vi "SDR_front_panel_V1.vi"() -> ()   [LabVIEW 2024]
uses:
  RPC Messages/rfcontrol_DeviceInformationResponse.ctl
  RPC Messages/rfcontrol_RFDC.ctl
  RPC Messages/rfcontrol_GetRFDCCenterFrequencyResponse.ctl
  RPC Messages/rfcontrol_GetRFDCGainResponse.ctl
  RPC Messages/rfcontrol_RFTile.ctl
  RPC Messages/rfcontrol_GetRFTileSampleRateResponse.ctl
  RPC Messages/rfcontrol_SetRFDCCenterFrequencyResponse.ctl
  RPC Messages/rfcontrol_SetRFDCGainResponse.ctl
  RPC Messages/rfcontrol_SetRFTileSampleRateResponse.ctl
  RPC Messages/rfcontrol_GetRFDCBackgroundCalibrationStateResponse.ctl
  RPC Messages/rfcontrol_SetRFDCBackgroundCalibrationStateResponse.ctl
  RPC Messages/rfcontrol_GetRFDCCalibrationBypassResponse.ctl
  RPC Messages/rfcontrol_SetRFDCCalibrationBypassResponse.ctl
  RPC Messages/rfcontrol_GetDeviceTempsResponse.ctl
  RPC Messages/rfcontrol_TemperatureReadings.ctl
  RPC Messages/rfcontrol_RFDCSendWaveformResponse.ctl
  FlexCompute_grpc_client/RPC Messages/rfcontrol_Response.ctl
  RPC Messages/rfcontrol_SetGPSUTCStartTimeResponse.ctl
  RPC Messages/rfcontrol_RFDCCaptureWaveformRequest.ctl
  RPC Messages/rfcontrol_DeviceInformationRequest.ctl
  RPC Messages/rfcontrol_RFDCSendWaveformRequest.ctl
  RPC Messages/rfcontrol_GetRFDCCenterFrequencyRequest.ctl
  RPC Messages/rfcontrol_GetRFDCGainRequest.ctl
  RPC Messages/rfcontrol_GetRFTileSampleRateRequest.ctl
  RPC Messages/rfcontrol_GetDeviceTempsRequest.ctl
  RPC Messages/rfcontrol_SetRFDCCenterFrequencyRequest.ctl
  RPC Messages/rfcontrol_SetRFDCGainRequest.ctl
  RPC Messages/rfcontrol_SetRFTileSampleRateRequest.ctl
  RPC Messages/rfcontrol_GetRFDCBackgroundCalibrationStateRequest.ctl
  RPC Messages/rfcontrol_SetRFDCBackgroundCalibrationStateRequest.ctl
  RPC Messages/rfcontrol_SetRFDCCalibrationBypassRequest.ctl
  RPC Messages/rfcontrol_GetRFDCCalibrationBypassRequest.ctl
  RPC Messages/rfcontrol_GetTriggerStatusRequest.ctl
  RPC Messages/rfcontrol_SetTriggerWaitRequest.ctl
  RPC Messages/rfcontrol_SetMaxTriggerLengthRequest.ctl
  RPC Messages/rfcontrol_ResetTriggerRequest.ctl
  RPC Messages/rfcontrol_StartGPSPollRequest.ctl
  RPC Messages/rfcontrol_StopGPSPollRequest.ctl
  RPC Messages/rfcontrol_SetGPSUTCStartTimeRequest.ctl
  FlexCompute_grpc_client/RPC Messages/rfcontrol_ControlParams.ctl
  FlexCompute_grpc_client/RPC Messages/rfcontrol_Empty.ctl
  RPC Messages/rfcontrol_GetGPSLastLocInfoRequest.ctl
  FlexSDR_gRPC_client.lvlib
  FlexCompute_grpc_client/FlexCompute_grpc_client.lvlib
panel:
  in  "FlexCompute Selection":u16(ring) items=["192.168.137.105:5555"]
  out "Error Out":errorcluster
  in  "Clear\nDevices":bool
  out "FlexSDR Search IP":string
  in  "FlexSDR Search Subnet":string
  in  "FlexSDR Selection":u16(ring) items=["192.168.137.76:5555", "192.168.137.105:5555", "192.168.137.173:5555", "192.168.137.174:5555"]
  in  "Scan for \nDevices":bool
  out "Hardware\nBusy":bool
  in  "Stop Program":bool
  in  "Main Container":T1(tab)
  in  "Set Default Scale":bool
  in  "Continuous I/Q Capture":bool
  in  "WFM Type":string(combo)
  in  "Send RFDC":T2
  in  "Set TX Waveform":bool
  out "Capture Error Status":i32
  out "Capture Error Message":string
  out "IQ Graph":cluster{"Y":dbl[], "Y":dbl[]}[](graph)
  in  "Capture Length":i32
  in  "Capture RFDC":T2
  in  "Single I/Q Capture":bool
  out "Send WFM Resp":T3
  out "FFT Mag":cluster{"Y":dbl[], "Y":dbl[]}[](graph)
  in  "Get Gain":bool
  in  "Gain RFDC":T2
  in  "Get Center\nFrequency":bool
  in  "Get Device\nInformation":bool
  out "Device\nInformation":T4
  in  "CF RFDC":T2
  out "Center Frequency Data":T5 {"center_frequency" format="%#_g MHz"}
  out "Gain Data":T6 {"gain" format="%#_g dB"}
  in  "Get Sample\nRate":bool
  in  "SR RFTile":T7
  out "Sample Rate Data":T8 {"sample_rate" format="%#_g MSps"}
  out "Device Temp Data":T9 {"temp_readings"."RPU_temp" format="%#_g °C"; "temp_readings"."APU_temp" format="%#_g °C"; "temp_readings"."PL_temp" format="%#_g °C"}
  in  "Get Temps":bool
  in  "Req SR":dbl format="%#_g MSps"
  in  "Set Sample\nRate":bool
  in  "SSR RFTile":T7
  in  "Set Gain":bool
  in  "SG RFDC":T2
  in  "Req Gain":dbl format="%#_g dB"
  in  "Set Center\nFrequency":bool
  in  "SCF RFDC":T2
  out "SCF Data":T11 {"center_frequency" format="%#_g MHz"}
  in  "Req CF":dbl format="%#_g MHz"
  out "SG Data":T12 {"gain" format="%#_g dB"}
  out "SSR Data":T13 {"sample_rate" format="%#_g MSps"}
  out "Analyzing\n100 MHz":bool
  out "Grabbing\n100 MHz":bool
  out "Analyzing\n400 MHz":bool
  out "Grabbing\n400 MHz":bool
  out "Analyzing\n1200 MHz":bool
  out "Grabbing\n1200 MHz":bool
  in  "Cal Level":dbl format="%#_g dBm"
  in  "Show Matlab":bool
  out "Writing \nCal Coeffs":bool
  out "100 EVM":dbl format="%#_g dB"
  out "400 EVM":dbl format="%#_g dB"
  out "1200 EVM":dbl format="%#_g dB"
  out "Complete":bool
  out "Analyzing\nFull BW":bool
  out "Grabbing\nFull BW":bool
  out "Cal FFT Mag":cluster{"Y":dbl[], "Y":dbl[]}[](graph)
  in  "Perform CAL":bool
  out "Full BW EVM":dbl format="%#_g dB"
  in  "New Cal Status":bool
  in  "SBCal RFDC":T2
  in  "Set Cal\nStatus":bool
  in  "Cal RFDC":T2
  in  "Get Cal\nStatus":bool
  in  "New Frozen\nStatus":bool
  in  "SBGCal RFDC":T2
  in  "Set BGCal\nStatus":bool
  in  "BGCal RFDC":T2
  in  "Get BGCal\nStatus":bool
  out "BGCal Data":T14
  out "SBGCal Data":T15
  out "Cal Status Data":T16
  out "SCal Status Data":T17
  out "Set Trig Max Length Error Status":i32
  out "Set Trig Max Length Error Message":string
  in  "Set Trig Max Length":bool
  out "Reset Trig Error Status":i32
  out "Reset Trig Error Message":string
  in  "Reset Trig":bool
  out "Set Trig Wait Error Status":i32
  out "Set Trig Wait Error Message":string
  in  "Set Hardware Trig":bool
  in  "Set Trig Max Length Value":i32 format="%.0f Samples"
  in  "Set Trig Delay":i32 format="%.0f Samples"
  in  "Set Trig Wait":bool
  out "Get Trig Status Error Status":i32
  out "Get Trig Status Error Message":string
  out "Hardware Trig?":bool
  out "Wait For Trig?":bool
  out "Triggered?":bool
  in  "Get Trig\nStatus":bool
  in  "Channel #":i32
  in  "Quad #":i32
  out "Trig Delay":i32 format="%.0f Samples"
  out "Trig Max Length":i32 format="%.0f Samples"
  in  "Display \nTimestamp?":bool
  in  "UTC Start Time":dbl format="%#_12g"
  in  "Set UTC\nStart Time":bool
  in  "GPS Num of Samples":i32(ring) items=["1 Sample"=1, "2 Samples"=2, "3 Samples"=3, "4 Samples"=4, "5 Samples"=5]
  out "GPS Poll Active":bool
  in  "Start GPS \nPoll":bool
  in  "Stop GPS\nPoll":bool
  in  "GPS Poll Time":dbl format="%#_g ms"
  out "GPS Actual Poll Time":u32 format="%.0f ms"
  out "GPS ECEF Y":dbl[](array[numeric]) format="%#_9g"
  out "GPS ECEF X":dbl[](array[numeric]) format="%#_9f"
  out "GPS ECEF Z":dbl[](array[numeric]) format="%#_9g"
  out "GPS error_status":i32
  out "GPS error_message":string
  out "GPS Time":string[](array[string])
  out "UTS Start Time Response":T18 {"utc_start_time" format="%#_12g"}
  in  "Set Peak Threshold":dbl format="%#_g dBm"
  in  "Update Server\nControls":bool
  out "KPI Error Message":string
  out "KPI Status":u32
  out "Mem Address":string
  out "Anomaly \nDetected":bool
  out "RSSI":dbl format="%#_g dBm"
  out "Actual KPI Poll Time":u32 format="%.0f ms"
  in  "KPI Poll":bool
  in  "KPI Poll Time":dbl format="%#_g ms"
  out "I Phase Rotation From Peak":dbl format="%#_g Hz"
  out "Peak Time Offset":dbl format="%#_g ns"
  out "Q Phase Rotation From Peak":dbl format="%#_g Hz"
  out "Peak Threshold":dbl format="%#_g dBm"
  out "Peak Time":dbl format="%#_g s"
  in  "Set Server Sample Rate":dbl format="%#_g MHz"
  in  "Set Carrier Frequency":dbl format="%#_g MHz"
  in  "Set Sync Length":i32 format="%.0f Samples"
  in  "Set Time Between Peaks":dbl format="%#_g µs"
  out "Update Server Controls Response":T19
  # "Tile Mapping:\n\nTXT1:\n1. TX1     2. TX2\n3. TX3     4. TX4\n\nTXT2:\n1. TX5     2. TX6\n3. TX7     4. TX8\n\nRXT1:\n1. RX1     2. RX2\n3. RX3     4. RX4\n\nRXT2:\n1. RX5     2. RX6\n3. RX7     4. RX8\n\nWRXT:\n1. WRX1   2.WRX2"
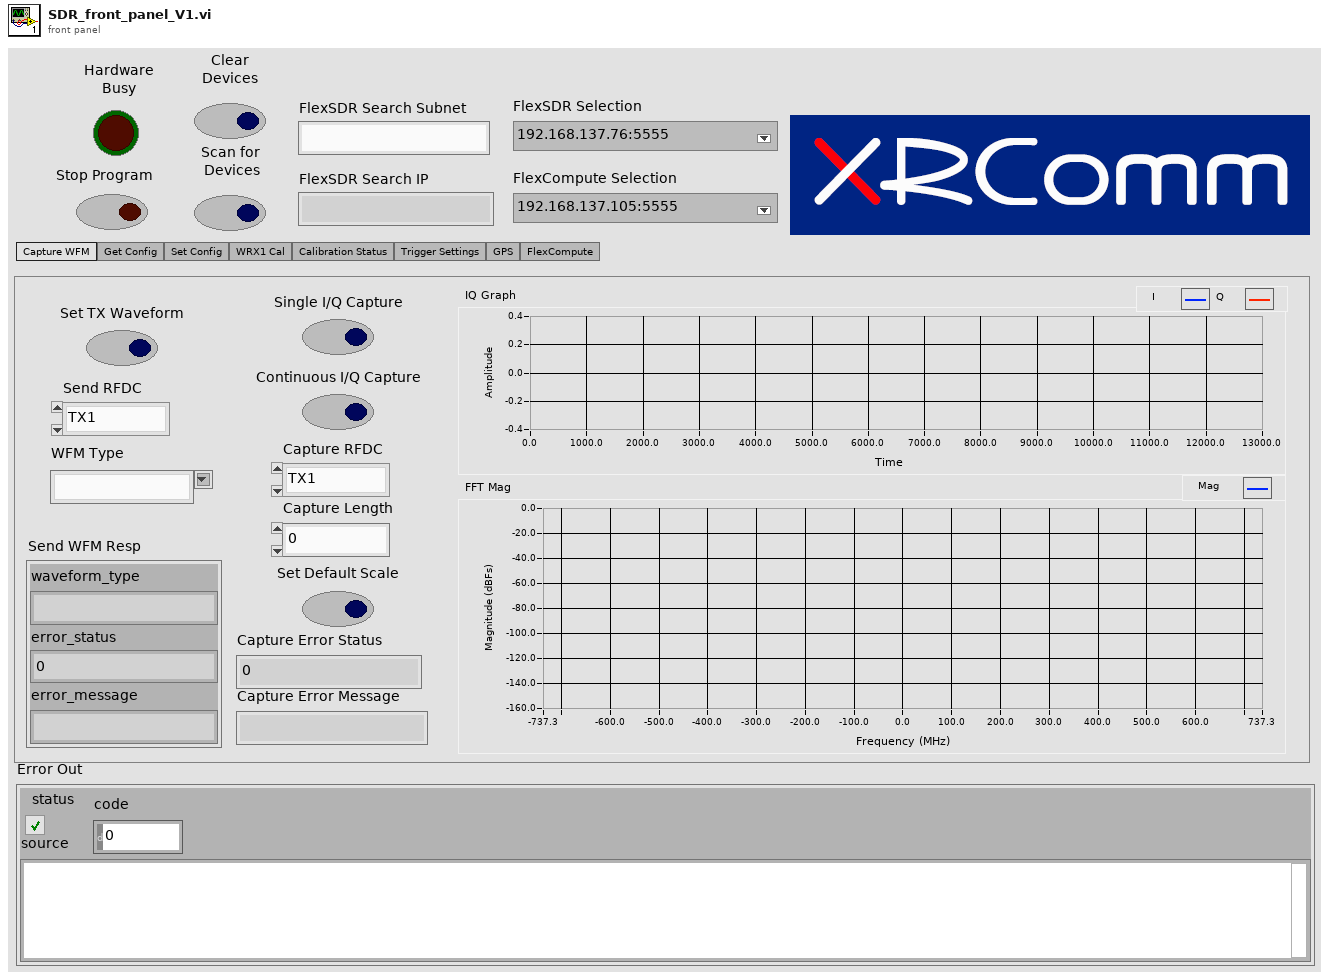
[diagram p1: front panel]
types:
  T1 = enum32{"Capture WFM", "Get Config", "Set Config", "WRX1 Cal", "Calibration Status", "Trigger Settings", "GPS", "FlexCompute"}
  T2 = typedef "FlexSDR_gRPC_client.lvlib/rfcontrol_RFDC.ctl" = enum32{"TX1", "TX2", "TX3", "TX4", "TX5", "TX6", "TX7", "TX8", "RX1", "RX2", "RX3", "RX4", "RX5", "RX6", "RX7", "RX8", "WRX1", "WRX2"}
  T3 = typedef "FlexSDR_gRPC_client.lvlib/rfcontrol_RFDCSendWaveformResponse.ctl" = cluster{"waveform_type":string, "error_status":i32, "error_message":string}
  T4 = typedef "FlexSDR_gRPC_client.lvlib/rfcontrol_DeviceInformationResponse.ctl" = cluster{"reply_information":string, "manufacturer":string, "model":string, "serial_number":i32, "firmware_revision":string}
  T5 = typedef "FlexSDR_gRPC_client.lvlib/rfcontrol_GetRFDCCenterFrequencyResponse.ctl" = cluster{"center_frequency":dbl, "error_status":i32, "error_message":string}
  T6 = typedef "FlexSDR_gRPC_client.lvlib/rfcontrol_GetRFDCGainResponse.ctl" = cluster{"gain":dbl, "error_status":i32, "error_message":string}
  T7 = typedef "FlexSDR_gRPC_client.lvlib/rfcontrol_RFTile.ctl" = enum32{"TXT1", "TXT2", "RXT1", "RXT2", "WRXT"}
  T8 = typedef "FlexSDR_gRPC_client.lvlib/rfcontrol_GetRFTileSampleRateResponse.ctl" = cluster{"sample_rate":dbl, "error_status":i32, "error_message":string}
  T9 = typedef "FlexSDR_gRPC_client.lvlib/rfcontrol_GetDeviceTempsResponse.ctl" = cluster{"temp_readings":T10, "error_status":i32, "error_message":string}
  T10 = typedef "FlexSDR_gRPC_client.lvlib/rfcontrol_TemperatureReadings.ctl" = cluster{"PL_temp":dbl, "APU_temp":dbl, "RPU_temp":dbl}
  T11 = typedef "FlexSDR_gRPC_client.lvlib/rfcontrol_SetRFDCCenterFrequencyResponse.ctl" = cluster{"center_frequency":dbl, "error_status":i32, "error_message":string}
  T12 = typedef "FlexSDR_gRPC_client.lvlib/rfcontrol_SetRFDCGainResponse.ctl" = cluster{"gain":dbl, "error_status":i32, "error_message":string}
  T13 = typedef "FlexSDR_gRPC_client.lvlib/rfcontrol_SetRFTileSampleRateResponse.ctl" = cluster{"sample_rate":dbl, "error_status":i32, "error_message":string}
  T14 = typedef "FlexSDR_gRPC_client.lvlib/rfcontrol_GetRFDCBackgroundCalibrationStateResponse.ctl" = cluster{"is_frozen":bool, "error_status":i32, "error_message":string}
  T15 = typedef "FlexSDR_gRPC_client.lvlib/rfcontrol_SetRFDCBackgroundCalibrationStateResponse.ctl" = cluster{"is_frozen":bool, "error_status":i32, "error_message":string}
  T16 = typedef "FlexSDR_gRPC_client.lvlib/rfcontrol_GetRFDCCalibrationBypassResponse.ctl" = cluster{"bypass_cal":bool, "error_status":i32, "error_message":string}
  T17 = typedef "FlexSDR_gRPC_client.lvlib/rfcontrol_SetRFDCCalibrationBypassResponse.ctl" = cluster{"bypass_cal":bool, "error_status":i32, "error_message":string}
  T18 = typedef "FlexSDR_gRPC_client.lvlib/rfcontrol_SetGPSUTCStartTimeResponse.ctl" = cluster{"utc_start_time":dbl, "error_status":i32, "error_message":string}
  T19 = typedef "FlexCompute_grpc_client.lvlib/rfcontrol_Response.ctl" = cluster{"message":string}
  T20 = enum8{"Enabled", "Disabled", "Disabled and Grayed Out"}
  T21 = typedef "FlexCompute_grpc_client.lvlib/rfcontrol_Empty.ctl" = cluster{"void":string}
  T22 = typedef "FlexSDR_gRPC_client.lvlib/rfcontrol_RFDCCaptureWaveformRequest.ctl" = cluster{"device_id":string, "rfdc":T2, "num_of_samples":i32, "error_queue_populate":bool}
  T23 = typedef "FlexSDR_gRPC_client.lvlib/rfcontrol_GetGPSLastLocInfoRequest.ctl" = cluster{"device_id":string, "num_of_samples":i32, "error_queue_populate":bool}
  T24 = typedef "FlexSDR_gRPC_client.lvlib/rfcontrol_DeviceInformationRequest.ctl" = cluster{"device_id":string, "error_queue_populate":bool}
  T25 = typedef "FlexSDR_gRPC_client.lvlib/rfcontrol_RFDCSendWaveformRequest.ctl" = cluster{"device_id":string, "rfdc":T2, "waveform_type":string, "error_queue_populate":bool}
  T26 = typedef "FlexSDR_gRPC_client.lvlib/rfcontrol_GetRFDCCenterFrequencyRequest.ctl" = cluster{"device_id":string, "rfdc":T2, "error_queue_populate":bool}
  T27 = typedef "FlexSDR_gRPC_client.lvlib/rfcontrol_GetRFDCGainRequest.ctl" = cluster{"device_id":string, "rfdc":T2, "error_queue_populate":bool}
  T28 = typedef "FlexSDR_gRPC_client.lvlib/rfcontrol_GetRFTileSampleRateRequest.ctl" = cluster{"device_id":string, "rftile":T7, "error_queue_populate":bool}
  T29 = typedef "FlexSDR_gRPC_client.lvlib/rfcontrol_GetDeviceTempsRequest.ctl" = cluster{"device_id":string, "error_queue_populate":bool}
  T30 = typedef "FlexSDR_gRPC_client.lvlib/rfcontrol_SetRFDCCenterFrequencyRequest.ctl" = cluster{"device_id":string, "rfdc":T2, "center_frequency":dbl, "error_queue_populate":bool}
  T31 = typedef "FlexSDR_gRPC_client.lvlib/rfcontrol_SetRFDCGainRequest.ctl" = cluster{"device_id":string, "rfdc":T2, "gain":dbl, "error_queue_populate":bool}
  T32 = typedef "FlexSDR_gRPC_client.lvlib/rfcontrol_SetRFTileSampleRateRequest.ctl" = cluster{"device_id":string, "rftile":T7, "sample_rate":dbl, "error_queue_populate":bool}
  T33 = typedef "FlexSDR_gRPC_client.lvlib/rfcontrol_SetRFDCCalibrationBypassRequest.ctl" = cluster{"device_id":string, "rfdc":T2, "bypass_cal":bool, "error_queue_populate":bool}
  T34 = typedef "FlexSDR_gRPC_client.lvlib/rfcontrol_SetRFDCBackgroundCalibrationStateRequest.ctl" = cluster{"device_id":string, "rfdc":T2, "is_frozen":bool, "error_queue_populate":bool}
  T35 = typedef "FlexSDR_gRPC_client.lvlib/rfcontrol_GetRFDCBackgroundCalibrationStateRequest.ctl" = cluster{"device_id":string, "rfdc":T2, "error_queue_populate":bool}
  T36 = typedef "FlexSDR_gRPC_client.lvlib/rfcontrol_GetRFDCCalibrationBypassRequest.ctl" = cluster{"device_id":string, "rfdc":T2, "error_queue_populate":bool}
  T37 = typedef "FlexSDR_gRPC_client.lvlib/rfcontrol_GetTriggerStatusRequest.ctl" = cluster{"device_id":string, "quad_num":i32, "channel_num":i32, "error_queue_populate":bool}
  T38 = typedef "FlexSDR_gRPC_client.lvlib/rfcontrol_SetTriggerWaitRequest.ctl" = cluster{"device_id":string, "quad_num":i32, "channel_num":i32, "trig_sample_delay":i32, "is_hardware_trig":bool, "error_queue_populate":bool}
  T39 = typedef "FlexSDR_gRPC_client.lvlib/rfcontrol_SetMaxTriggerLengthRequest.ctl" = cluster{"device_id":string, "quad_num":i32, "channel_num":i32, "max_trig_length":i32, "error_queue_populate":bool}
  T40 = typedef "FlexSDR_gRPC_client.lvlib/rfcontrol_ResetTriggerRequest.ctl" = cluster{"device_id":string, "quad_num":i32, "channel_num":i32, "error_queue_populate":bool}
  T41 = typedef "FlexSDR_gRPC_client.lvlib/rfcontrol_StartGPSPollRequest.ctl" = cluster{"device_id":string, "error_queue_populate":bool}
  T42 = typedef "FlexSDR_gRPC_client.lvlib/rfcontrol_StopGPSPollRequest.ctl" = cluster{"device_id":string, "error_queue_populate":bool}
  T43 = typedef "FlexSDR_gRPC_client.lvlib/rfcontrol_SetGPSUTCStartTimeRequest.ctl" = cluster{"device_id":string, "utc_start_time":dbl, "error_queue_populate":bool}
  T44 = typedef "FlexCompute_grpc_client.lvlib/rfcontrol_ControlParams.ctl" = cluster{"peak_threshold":dbl, "sampling_rate_hz":dbl, "carrier_frequency_hz":dbl, "sync_length_samples":u32, "time_between_peaks_s":dbl}
  T45 = typedef "grpc-lvsupport-release.lvlib/grpcId.ctl" = u64
  T46 = typedef "FlexSDR_gRPC_client.lvlib/rfcontrol_RFDCCaptureWaveformResponse.ctl" = cluster{"I":dbl[], "Q":dbl[], "error_status":i32, "error_message":string}
  T47 = typedef "FlexSDR_gRPC_client.lvlib/rfcontrol_GetTriggerStatusResponse.ctl" = cluster{"quad_num":i32, "channel_num":i32, "triggered":bool, "wait_for_trig":bool, "trig_sample_delay":i32, "is_hardware_trig":bool, "max_trig_length":i32, "error_status":i32, "error_message":string}
  T48 = typedef "FlexSDR_gRPC_client.lvlib/rfcontrol_SetTriggerWaitResponse.ctl" = cluster{"quad_num":i32, "channel_num":i32, "trig_sample_delay":i32, "is_hardware_trig":bool, "error_status":i32, "error_message":string}
  T49 = typedef "FlexSDR_gRPC_client.lvlib/rfcontrol_SetMaxTriggerLengthResponse.ctl" = cluster{"quad_num":i32, "channel_num":i32, "max_trig_length":i32, "error_status":i32, "error_message":string}
  T50 = typedef "FlexSDR_gRPC_client.lvlib/rfcontrol_ResetTriggerResponse.ctl" = cluster{"quad_num":i32, "channel_num":i32, "error_status":i32, "error_message":string}
  T51 = typedef "FlexSDR_gRPC_client.lvlib/rfcontrol_StartGPSPollResponse.ctl" = cluster{"gps_poll_status":bool, "error_status":i32, "error_message":string}
  T52 = typedef "FlexSDR_gRPC_client.lvlib/rfcontrol_StopGPSPollResponse.ctl" = cluster{"gps_poll_status":bool, "error_status":i32, "error_message":string}
  T53 = typedef "FlexSDR_gRPC_client.lvlib/rfcontrol_GetGPSLastLocInfoResponse.ctl" = cluster{"time":dbl[], "ecef_x":dbl[], "ecef_y":dbl[], "ecef_z":dbl[], "error_status":i32, "error_message":string}
  T54 = typedef "FlexCompute_grpc_client.lvlib/rfcontrol_KPIData.ctl" = cluster{"peak_threshold":dbl, "rssi_db":dbl, "timing_offset_s":dbl, "peak_index_samples":i32, "peak_time_s":dbl, "is_anomaly":bool, "mem_address":string, "status":T55, "error_message":string, "phase_rotation_from_peak_I":sgl, "phase_rotation_from_peak_Q":sgl}
  T55 = typedef "FlexCompute_grpc_client.lvlib/rfcontrol_Status.ctl" = enum32{"SUCCESS", "ERROR"}
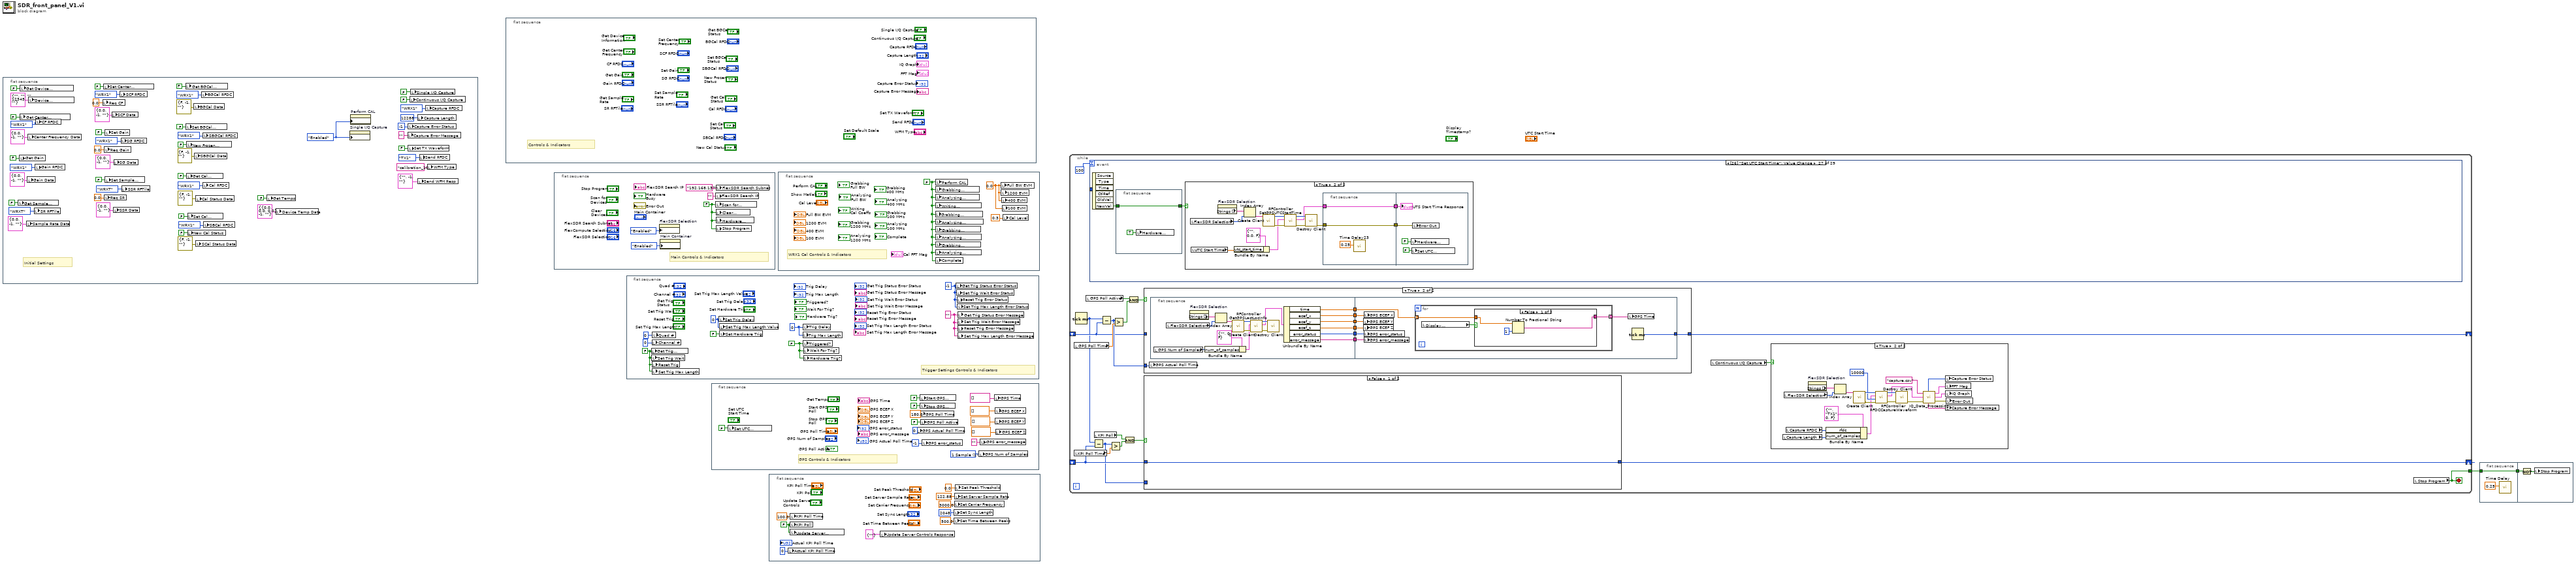
[diagram p0: block diagram]
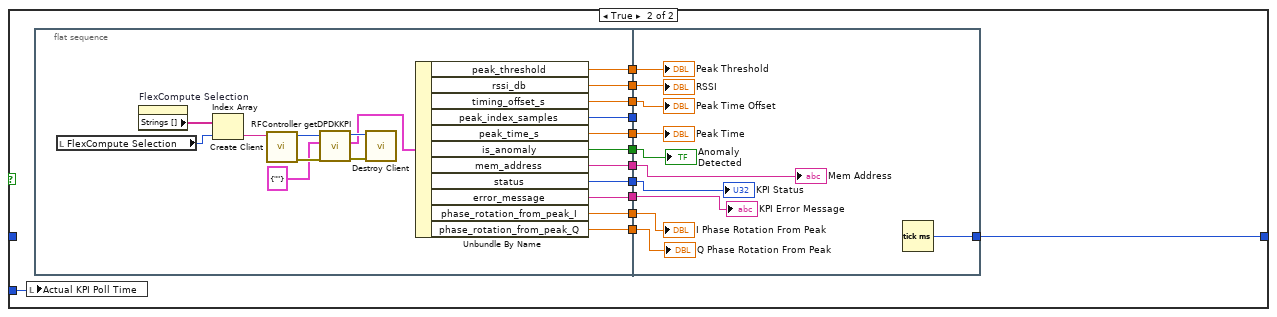
[diagram p2: hidden frame]
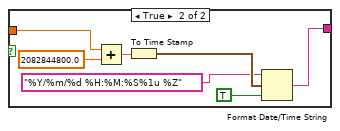
[diagram p5: hidden frame]
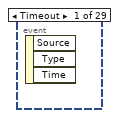
[diagram p6: hidden frame]
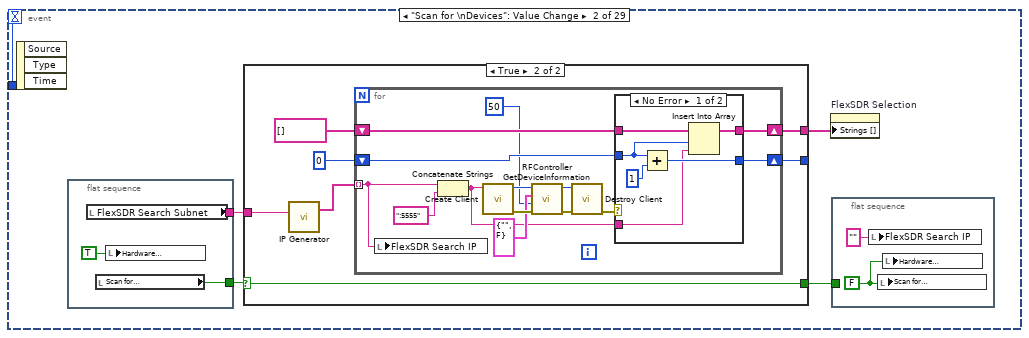
[diagram p7: hidden frame]
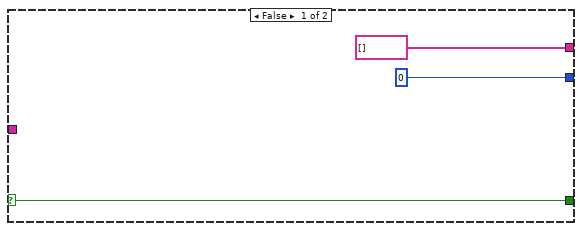
[diagram p8: hidden frame]
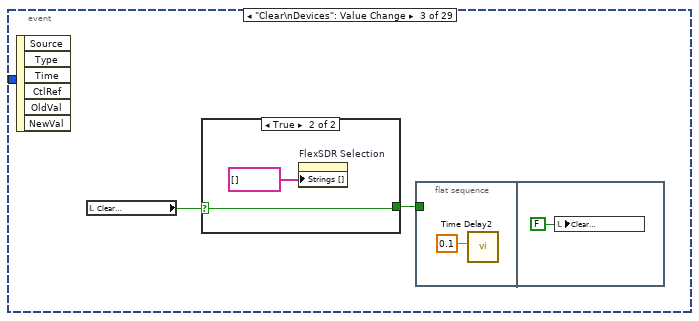
[diagram p10: hidden frame]
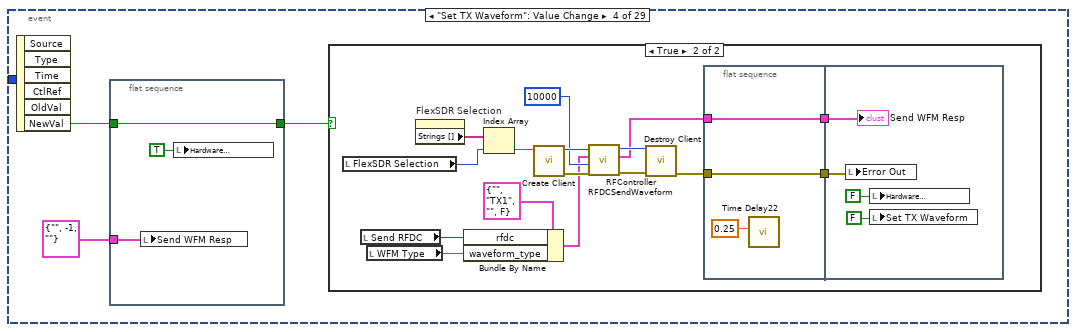
[diagram p12: hidden frame]
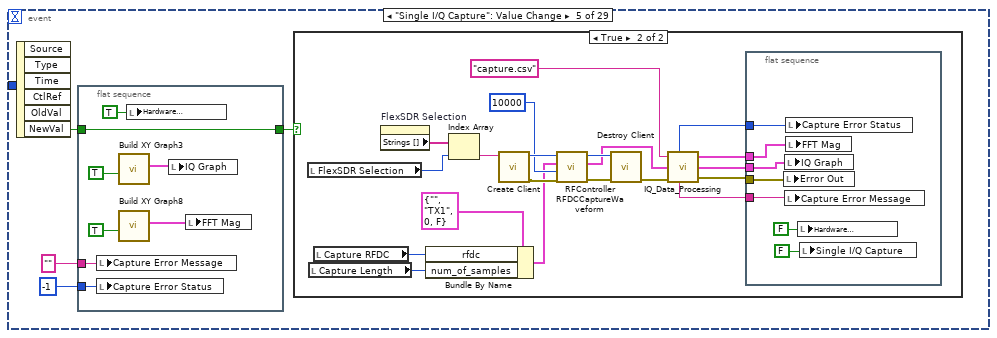
[diagram p14: hidden frame]
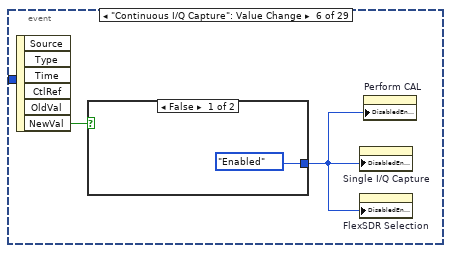
[diagram p16: hidden frame]
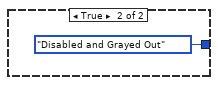
[diagram p17: hidden frame]
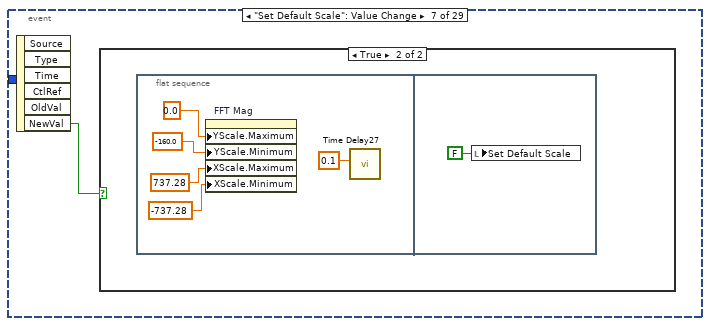
[diagram p18: hidden frame]
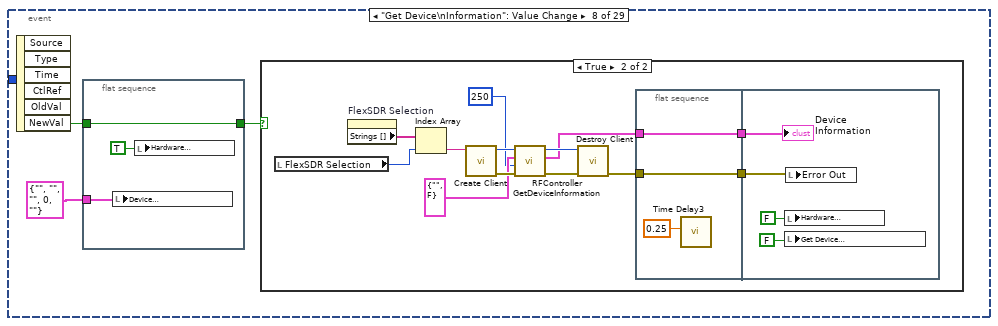
[diagram p20: hidden frame]
diagram:
  n1 = flat-sequence {
    frame #0 {
      w3 = T20."Enabled" ("Disabled")
      # "Initial Settings"
      n2 = local write "Get Sample\nRate"(FALSE ("Get Sample\nRate")) -> ()
      n3 = local write "Get Gain"(FALSE ("Get Gain")) -> ()
      n4 = local write "Get Center\nFrequency"(FALSE ("Get Center\nFrequency")) -> ()
      n5 = local write "Get Device\nInformation"(FALSE ("Get Device\nInformation")) -> ()
      n6 = local write "Sample Rate Data"(T8 {"sample_rate"=0.0, "error_status"=-1, "error_message"=""} ("Sample Rate Data")) -> ()
      n7 = local write "Gain Data"(T6 {"gain"=0.0, "error_status"=-1, "error_message"=""} ("Gain Data")) -> ()
      n8 = local write "Center Frequency Data"(T5 {"center_frequency"=0.0, "error_status"=-1, "error_message"=""} ("Center Frequency Data")) -> ()
      n9 = local write "Device\nInformation"(T4 {"reply_information"="", "manufacturer"="", "model"="", "serial_number"=12345, "firmware_revision"=""} ("Device\nInformation")) -> ()
      n10 = local write "SR RFTile"(rfcontrol_RFTile."WRXT" ("SR RFTile")) -> ()
      n11 = local write "Gain RFDC"(rfcontrol_RFDC."WRX1" ("Gain RFDC")) -> ()
      n12 = local write "CF RFDC"(rfcontrol_RFDC."WRX1" ("CF RFDC")) -> ()
      n13 = local write "Req CF"(0.0 ("Req CF")) -> ()
      n14 = local write "Set Center\nFrequency"(FALSE ("Set Center\nFrequency")) -> ()
      n15 = local write "Req Gain"(0.0 ("Req Gain")) -> ()
      n16 = local write "Req SR"(0.0 ("Req SR")) -> ()
      n17 = local write "Set Gain"(FALSE ("Set Gain")) -> ()
      n18 = local write "Set Sample\nRate"(FALSE ("Set Sample\nRate")) -> ()
      n19 = local write "SCF Data"(T11 {"center_frequency"=0.0, "error_status"=-1, "error_message"=""} ("Response Data")) -> ()
      n20 = local write "SSR Data"(T13 {"sample_rate"=0.0, "error_status"=-1, "error_message"=""} ("SSR Data")) -> ()
      n21 = local write "SG Data"(T12 {"gain"=0.0, "error_status"=-1, "error_message"=""} ("SG Data")) -> ()
      n22 = local write "SCF RFDC"(rfcontrol_RFDC."WRX1" ("SCF RFDC")) -> ()
      n23 = local write "SG RFDC"(rfcontrol_RFDC."WRX1" ("SG RFDC")) -> ()
      n24 = local write "SSR RFTile"(rfcontrol_RFTile."WRXT" ("SSR Tile")) -> ()
      n25 = local write "Get BGCal\nStatus"(FALSE ("Get BGCal\nStatus")) -> ()
      n26 = local write "Set BGCal\nStatus"(FALSE ("Set BGCal\nStatus")) -> ()
      n27 = local write "New Frozen\nStatus"(FALSE ("New Frozen\nStatus")) -> ()
      n28 = local write "Get Cal\nStatus"(FALSE ("Get Cal\nStatus")) -> ()
      n29 = local write "Set Cal\nStatus"(FALSE ("Set Cal\nStatus")) -> ()
      n30 = local write "New Cal Status"(FALSE ("New Cal Status")) -> ()
      n31 = local write "BGCal Data"(T14 {"is_frozen"=FALSE, "error_status"=-1, "error_message"=""} ("BGCal Data")) -> ()
      n32 = local write "SBGCal Data"(T15 {"is_frozen"=FALSE, "error_status"=-1, "error_message"=""} ("SBGCal Data")) -> ()
      n33 = local write "SCal Status Data"(T17 {"bypass_cal"=FALSE, "error_status"=-1, "error_message"=""} ("SCal Status Data")) -> ()
      n34 = local write "Cal Status Data"(T16 {"bypass_cal"=FALSE, "error_status"=-1, "error_message"=""} ("Cal Status Data")) -> ()
      n35 = local write "BGCal RFDC"(rfcontrol_RFDC."WRX1" ("BGCal RFDC")) -> ()
      n36 = local write "SBGCal RFDC"(rfcontrol_RFDC."WRX1" ("SBGCal RFDC")) -> ()
      n37 = local write "Cal RFDC"(rfcontrol_RFDC."WRX1" ("Cal RFDC")) -> ()
      n38 = local write "SBCal RFDC"(rfcontrol_RFDC."WRX1" ("SBCal RFDC")) -> ()
      n39 = local write "Get Temps"(FALSE ("Get Temps")) -> ()
      n40 = local write "Device Temp Data"(T9 {"temp_readings"={"PL_temp"=0.0, "APU_temp"=0.0, "RPU_temp"=0.0}, "error_status"=-1, "error_message"=""} ("Device Temp Data")) -> ()
      n41 = property on="Single I/Q Capture" class="Bool (strict)"("DisabledEnum"=w3) -> ()  [unwired: 2 in, 2 out]
      n42 = property on="Perform CAL" class="Bool (strict)"("DisabledEnum"=w3) -> ()  [unwired: 2 in, 2 out]
      n43 = local write "Capture Error Message"("" ("Capture Error Message")) -> ()
      n44 = local write "Capture Error Status"(-1 ("Capture Error Status")) -> ()
      n45 = local write "Set TX Waveform"(FALSE ("Set TX Waveform")) -> ()
      n46 = local write "Continuous I/Q Capture"(FALSE ("Continuous I/Q Capture")) -> ()
      n47 = local write "Single I/Q Capture"(FALSE ("Grab I/Q Waveform")) -> ()
      n48 = local write "Capture Length"(12288 ("Capture Length")) -> ()
      n49 = local write "Send WFM Resp"(T3 {"waveform_type"="", "error_status"=-1, "error_message"=""} ("Send WFM Resp")) -> ()
      n50 = local write "Send RFDC"(rfcontrol_RFDC."TX1" ("Send RFDC")) -> ()
      n51 = local write "Capture RFDC"(rfcontrol_RFDC."WRX1" ("Capture RFDC")) -> ()
      n52 = local write "WFM Type"("calibration_100" ("WFM Type")) -> ()
    }
  }
  n53 = flat-sequence {
    frame #0 {
      # "Controls & Indicators"
    }
  }
  n54 = flat-sequence {
    frame #0 {
      w55 = FALSE ("Scan for \nDevices")
      # "Main Controls & Indicators"
      n55 = property on="FlexSDR Selection" class="Ring (strict)"("DisabledEnum"=T20."Enabled" ("Disabled")) -> ()  [unwired: 2 in, 2 out]
      n56 = property on="Main Container" class="TabCtl (strict)"("DisabledEnum"=T20."Enabled" ("Disabled")) -> ()  [unwired: 2 in, 2 out]
      n57 = local write "FlexSDR Search IP"("" ("Current Search IP")) -> ()
      n58 = local write "Scan for \nDevices"(w55) -> ()
      n59 = local write "FlexSDR Search Subnet"("192.168.137" ("Search Subnet")) -> ()
      n60 = local write "Clear\nDevices"(w55) -> ()
      n61 = local write "Hardware\nBusy"(w55) -> ()
      n62 = local write "Stop Program"(w55) -> ()
    }
  }
  n63 = flat-sequence {
    frame #0 {
      w60 = "" ("Set Trig Wait Error Message")
      w61 = -1 ("Set Trig Wait Error Status")
      w59 = 0 ("Set Trig Delay")
      w63 = 0 ("Trig Delay")
      w64 = FALSE ("Triggered?")
      w58 = FALSE ("Get Trig\nStatus")
      # "Trigger Settings Controls & Indicators"
      n64 = local write "Get Trig\nStatus"(w58) -> ()
      n65 = local write "Set Trig Wait"(w58) -> ()
      n66 = local write "Channel #"(0 ("Channel #")) -> ()
      n67 = local write "Reset Trig"(w58) -> ()
      n68 = local write "Set Trig Max Length"(w58) -> ()
      n69 = local write "Quad #"(0 ("Quad #")) -> ()
      n70 = local write "Set Trig Delay"(w59) -> ()
      n71 = local write "Set Trig Max Length Value"(w59) -> ()
      n72 = local write "Set Hardware Trig"(FALSE ("Set Hardware Trig")) -> ()
      n73 = local write "Trig Max Length"(w63) -> ()
      n74 = local write "Trig Delay"(w63) -> ()
      n75 = local write "Triggered?"(w64) -> ()
      n76 = local write "Wait For Trig?"(w64) -> ()
      n77 = local write "Hardware Trig?"(w64) -> ()
      n78 = local write "Get Trig Status Error Status"(w61) -> ()
      n79 = local write "Set Trig Wait Error Status"(w61) -> ()
      n80 = local write "Reset Trig Error Status"(w61) -> ()
      n81 = local write "Set Trig Max Length Error Status"(w61) -> ()
      n82 = local write "Get Trig Status Error Message"(w60) -> ()
      n83 = local write "Set Trig Wait Error Message"(w60) -> ()
      n84 = local write "Reset Trig Error Message"(w60) -> ()
      n85 = local write "Set Trig Max Length Error Message"(w60) -> ()
    }
  }
  n86 = flat-sequence {
    frame #0 {
      w68 = 1 items=["1 Sample"=1, "2 Samples"=2, "3 Samples"=3, "4 Samples"=4, "5 Samples"=5] ("GPS Num of Samples")
      # "GPS Controls & Indicators"
      n87 = local write "Set UTC\nStart Time"(FALSE ("Set UTC\nStart Time")) -> ()
      n88 = local write "GPS Actual Poll Time"(u32 0 ("Actual Poll Time")) -> ()
      n89 = local write "GPS Poll Time"(180.0 ("Poll Time")) -> ()
      n90 = local write "Start GPS \nPoll"(FALSE ("Start GPS \nPoll")) -> ()
      n91 = local write "Stop GPS\nPoll"(FALSE ("Stop GPS\nPoll")) -> ()
      n92 = local write "GPS Poll Active"(FALSE ("GPS Poll Active")) -> ()
      n93 = local write "GPS error_status"(-1 ("GPS error_status")) -> ()
      n94 = local write "GPS Num of Samples"(w68) -> ()
      n95 = local write "GPS error_message"("" ("GPS error_message")) -> ()
      n96 = local write "GPS Time"(string[] [] ("GPS Time")) -> ()
      n97 = local write "GPS ECEF X"(dbl[] [] ("ecef_x")) -> ()
      n98 = local write "GPS ECEF Y"(dbl[] [] ("ecef_y")) -> ()
      n99 = local write "GPS ECEF Z"(dbl[] [] ("ecef_z")) -> ()
    }
  }
  n100 = flat-sequence {
    frame #0 {
      w86 = FALSE ("KPI Poll")
      n101 = local write "Actual KPI Poll Time"(u32 0 ("Actual KPI Poll Time")) -> ()
      n102 = local write "KPI Poll Time"(100.0 ("KPI Poll Time")) -> ()
      n103 = local write "KPI Poll"(w86) -> ()
      n104 = local write "Update Server\nControls"(w86) -> ()
      n105 = local write "Update Server Controls Response"(T19 {"message"=""} ("Update Server Controls Response")) -> ()
      n106 = local write "Set Sync Length"(2048 ("Set Sync Length")) -> ()
      n107 = local write "Set Time Between Peaks"(500.0 ("Set Time Between Peaks")) -> ()
      n108 = local write "Set Carrier Frequency"(3000.0 ("Set Carrier Frequency")) -> ()
      n109 = local write "Set Server Sample Rate"(122.88 ("Set Server Sample Rate")) -> ()
      n110 = local write "Set Peak Threshold"(0.0 ("Set Peak Threshold")) -> ()
    }
  }
  n111 = flat-sequence {
    frame #0 {
      w89 = FALSE ("Get Cal WFM")
      w91 = 0.0 ("Full BW EVM")
      # "WRX1 Cal Controls & Indicators"
      n112 = local write "Grabbing\n1200 MHz"(w89) -> ()
      n113 = local write "Perform CAL"(w89) -> ()
      n114 = local write "Grabbing\nFull BW"(w89) -> ()
      n115 = local write "Analyzing\nFull BW"(w89) -> ()
      n116 = local write "Writing \nCal Coeffs"(w89) -> ()
      n117 = local write "Analyzing\n1200 MHz"(w89) -> ()
      n118 = local write "Grabbing\n400 MHz"(w89) -> ()
      n119 = local write "Analyzing\n400 MHz"(w89) -> ()
      n120 = local write "Grabbing\n100 MHz"(w89) -> ()
      n121 = local write "Analyzing\n100 MHz"(w89) -> ()
      n122 = local write "Complete"(w89) -> ()
      n123 = local write "Full BW EVM"(w91) -> ()
      n124 = local write "1200 EVM"(w91) -> ()
      n125 = local write "400 EVM"(w91) -> ()
      n126 = local write "100 EVM"(w91) -> ()
      n127 = local write "Cal Level"(0.3 ("Cal Level")) -> ()
    }
  }
  n128 = while {
    tunnel: [w109] -> w2
    shift-right: [w107] -> _
    shift-left: _ -> [w101]
    shift-right: [w94] -> _
    shift-left: _ -> [w93]
    stop <- w109 stop-if-true
    n129 = local read "KPI Poll Time"() -> (w98:dbl)
    n130 = local read "GPS Poll Time"() -> (w105:dbl)
    n131 = Tick Count (ms)() -> (millisecond timer value=w99:u32)
    n132 = local read "GPS Poll Active"() -> (w106:bool)
    n133 = event shown="[26] \"Set UTC Start Time\": Value Change" {
      selector: _ -> [_ _ _ _ _ _ _ _ _ _ _ _ _ _ _ _ _ _ _ _ _ _ _ _ _ _ _ _ _]
      dyn-events: _ -> [_ _ _ _ _ _ _ _ _ _ _ _ _ _ _ _ _ _ _ _ _ _ _ _ _ _ _ _ _]
      timeout: 100 -> [_ w225 _ _ _ _ _ _ _ _ _ _ _ _ _ _ _ _ _ _ _ _ _ _ _ _ _ _ _]
      tunnel: [_ w225 _ _ _ _ _ _ _ _ _ _ _ _ _ _ _ _ _ _ _ _ _ _ _ _ _ _ _] -> _
      event Timeout {
        n134 = event-data() -> ()  [unwired: 1 in, 3 out]
      }
      event "Scan for \nDevices": Value Change {
        n135 = event-data() -> ()  [unwired: 1 in, 3 out]
        n136 = flat-sequence {
          tunnel: [w229] -> w226
          tunnel: [w228] -> w223
          frame #0 {
            n137 = local read "FlexSDR Search Subnet"() -> (w228:string)
            n138 = local read "Scan for \nDevices"() -> (w229:bool)
            n139 = local write "Hardware\nBusy"(TRUE ("Hardware\nBusy")) -> ()
          }
        }
        n140 = case shown="True" w226 {
          selector: w226 -> [w234 w240]
          tunnel: w223 -> [_ w241]
          tunnel: [w234 w240] -> w224
          tunnel: [string[] [] w237] -> w222
          tunnel: [0 w236] -> _
          frame False {
          }
          frame True {
            n141 = call "IP Generator.vi"("String"=w241) -> ("Array"=w235:string[])  [unwired: 2 in]
            n142 = for {
              tunnel: w235 -> [w242] mode=indexing
              shift-right: [w252] -> w236
              shift-left: 0 -> [w253]
              shift-right: [w251] -> w237
              shift-left: string[] [] -> [w254]
              n143 = local write "FlexSDR Search IP"(w242) -> ()
              n144 = Concatenate Strings(w242, ":5555" ("string")) -> (w244:string)
              n145 = call "Create Client.vi"("address"=w244) -> ("error out"=w250:errorcluster, "gRPC ID Out"=w248:T45)  [unwired: 9 in]
              n146 = call "RFController GetDeviceInformation.vi"("error in"=w250, "timeout (ms)"=50, "Request Data"=T24 {"device_id"="", "error_queue_populate"=FALSE}, "gRPC ID"=w248) -> ("error out"=w247:errorcluster, "gRPC ID out"=w246:T45)  [unwired: 5 in, 1 out]
              n147 = call "Destroy Client.vi"("error in"=w247, "gRPC ID"=w246) -> ("error out"=w243:errorcluster)  [unwired: 9 in]
              n148 = case shown="No Error" w243 {
                tunnel: w254 -> [w258 w262]
                tunnel: w253 -> [w259 w263]
                tunnel: [w260 w263] -> w252
                tunnel: w244 -> [w257 _]
                tunnel: [w256 w262] -> w251
                frame No Error {
                  n149 = Add(x=w259, y=1) -> (x+y=w260:i32)
                  n150 = Insert Into Array(array=w258, index=w259, new element=w257) -> (w256:string[])
                }
                frame Error {
                }
              }
            }
          }
        }
        n151 = property on="FlexSDR Selection" class="Ring (strict)"("Strings []"=w222) -> ()  [unwired: 2 in, 2 out]
        n152 = flat-sequence {
          tunnel: w224 -> [_]
          frame #0 {
            w231 = FALSE ("Scan for \nDevices")
            n153 = local write "FlexSDR Search IP"("" ("Current Search IP")) -> ()
            n154 = local write "Scan for \nDevices"(w231) -> ()
            n155 = local write "Hardware\nBusy"(w231) -> ()
          }
        }
      }
      event "Clear\nDevices": Value Change {
        n156 = event-data() -> ()  [unwired: 1 in, 6 out]
        n157 = local read "Clear\nDevices"() -> (w265:bool)
        n158 = case shown="True" w265 {
          selector: w265 -> [w268 w269]
          tunnel: [w268 w269] -> w264
          frame False {
          }
          frame True {
            n159 = property on="FlexSDR Selection" class="Ring (strict)"("Strings []"=string[] []) -> ()  [unwired: 2 in, 2 out]
          }
        }
        n160 = flat-sequence {
          tunnel: w264 -> [_]
          frame #0 {
            n161 = call "Time Delay2"("Delay Time (s)"=0.1) -> ()  [unwired: 10 in, 1 out]
          }
          frame #1 {
            n162 = local write "Clear\nDevices"(FALSE ("Clear\nDevices")) -> ()
          }
        }
      }
      event "Set TX Waveform": Value Change {
        n163 = event-data() -> ("NewVal"=w273:bool)  [unwired: 1 in, 5 out]
        n164 = flat-sequence {
          tunnel: w273 -> [w276]
          tunnel: [w276] -> w272
          tunnel: T3 {"waveform_type"="", "error_status"=-1, "error_message"=""} ("Send WFM Resp") -> [w274]
          frame #0 {
            n165 = local write "Send WFM Resp"(w274) -> ()
            n166 = local write "Hardware\nBusy"(TRUE ("Hardware\nBusy")) -> ()
          }
        }
        n167 = case shown="True" w272 {
          frame False {
          }
          frame True {
            n168 = local read "FlexSDR Selection"() -> (w291:u16)
            n169 = local read "Send RFDC"() -> (w281:T2)
            n170 = local read "WFM Type"() -> (w280:string)
            n171 = property on="FlexSDR Selection" class="Ring (strict)"() -> ("Strings []"=w292:string[])  [unwired: 2 in, 2 out]
            n172 = Bundle By Name(cluster=T25 {"device_id"="", "rfdc"=enum."TX1", "waveform_type"="", "error_queue_populate"=FALSE} ("Request Data"), "rfdc"=w281, "waveform_type"=w280) -> (w279:T25)
            n173 = Index Array(array=w292, index=w291) -> (element=w289:string)
            n174 = call "Create Client.vi"("address"=w289) -> ("error out"=w287:errorcluster, "gRPC ID Out"=w285:T45)  [unwired: 9 in]
            n175 = call "RFController RFDCSendWaveform.vi"("error in"=w287, "timeout (ms)"=10000, "Request Data"=w279, "gRPC ID"=w285) -> ("error out"=w286:errorcluster, "Response Data"=w277:T3, "gRPC ID out"=w284:T45)  [unwired: 5 in]
            n176 = call "Destroy Client.vi"("error in"=w286, "gRPC ID"=w284) -> ("error out"=w290:errorcluster)  [unwired: 9 in]
            n177 = flat-sequence {
              tunnel: w290 -> [w294]
              tunnel: [w294] -> w288
              tunnel: [w293] -> w278
              tunnel: w277 -> [w293]
              tunnel: w288 -> [w297]
              tunnel: w278 -> [w296]
              frame #0 {
                n178 = call "Time Delay22"("Delay Time (s)"=0.25) -> ()  [unwired: 10 in, 1 out]
              }
              frame #1 {
                n179 = local write "Error Out"(w297) -> ()
                n180 = local write "Hardware\nBusy"(FALSE ("Hardware\nBusy")) -> ()
                n181 = local write "Set TX Waveform"(FALSE ("Get Device\nInformation")) -> ()
                "Send WFM Resp" <- w296
              }
            }
          }
        }
      }
      event "Single I/Q Capture": Value Change {
        n182 = event-data() -> ("NewVal"=w303:bool)  [unwired: 1 in, 5 out]
        n183 = flat-sequence {
          tunnel: w303 -> [w311]
          tunnel: [w311] -> w302
          tunnel: "" ("Capture Error Message") -> [w307]
          tunnel: -1 ("Capture Error Status") -> [w306]
          frame #0 {
            n184 = local write "Capture Error Message"(w307) -> ()
            n185 = local write "Capture Error Status"(w306) -> ()
            n186 = call "Build XY Graph3"("Reset"=TRUE) -> ("XY Graph"=w309:cluster{"X":dbl[], "Y":dbl[]}[])  [unwired: 9 in, 1 out]
            n187 = call "Build XY Graph8"("Reset"=TRUE) -> ("XY Graph"=w304:cluster{"X":dbl[], "Y":dbl[]}[])  [unwired: 9 in, 1 out]
            n188 = local write "Hardware\nBusy"(TRUE ("Hardware\nBusy")) -> ()
            n189 = local write "IQ Graph"(w309) -> ()
            n190 = local write "FFT Mag"(w304) -> ()
          }
        }
        n191 = case shown="True" w302 {
          frame False {
          }
          frame True {
            n192 = local read "FlexSDR Selection"() -> (w330:u16)
            n193 = local read "Capture Length"() -> (w321:i32)
            n194 = local read "Capture RFDC"() -> (w328:T2)
            n195 = property on="FlexSDR Selection" class="Ring (strict)"() -> ("Strings []"=w331:string[])  [unwired: 2 in, 2 out]
            n196 = Bundle By Name(cluster=T22 {"device_id"="", "rfdc"=enum."TX1", "num_of_samples"=0, "error_queue_populate"=FALSE} ("Request Data"), "rfdc"=w328, "num_of_samples"=w321) -> (w320:T22)
            n197 = Index Array(array=w331, index=w330) -> (element=w329:string)
            n198 = call "Create Client.vi"("address"=w329) -> ("error out"=w327:errorcluster, "gRPC ID Out"=w326:T45)  [unwired: 9 in]
            n199 = call "RFController RFDCCaptureWaveform.vi"("error in"=w327, "timeout (ms)"=10000, "Request Data"=w320, "gRPC ID"=w326) -> ("error out"=w325:errorcluster, "Response Data"=w317:T46, "gRPC ID out"=w324:T45)  [unwired: 5 in]
            n200 = call "Destroy Client.vi"("error in"=w325, "gRPC ID"=w324) -> ("error out"=w319:errorcluster)  [unwired: 9 in]
            n201 = call "IQ_Data_Processing.vi"("file name"="capture.csv", "WFM Capture Response"=w317, "error in"=w319) -> ("gRPC error_status"=w316:i32, "gRPC error_message"=w312:string, "FFT Mag XY"=w313:cluster{"X":dbl[], "Y":dbl[]}[], "IQ XY"=w314:cluster{"X":dbl[], "Y":dbl[]}[], "error out"=w315:errorcluster)
            n202 = flat-sequence {
              tunnel: w315 -> [w336]
              tunnel: w316 -> [w333]
              tunnel: w314 -> [w335]
              tunnel: w313 -> [w334]
              tunnel: w312 -> [w332]
              frame #0 {
                n203 = local write "Error Out"(w336) -> ()
                n204 = local write "IQ Graph"(w335) -> ()
                n205 = local write "Capture Error Message"(w332) -> ()
                n206 = local write "Capture Error Status"(w333) -> ()
                n207 = local write "FFT Mag"(w334) -> ()
                n208 = local write "Hardware\nBusy"(FALSE ("Hardware\nBusy")) -> ()
                n209 = local write "Single I/Q Capture"(FALSE ("Get Device\nInformation")) -> ()
              }
            }
          }
        }
      }
      event "Continuous I/Q Capture": Value Change {
        n210 = event-data() -> ("NewVal"=w340:bool)  [unwired: 1 in, 5 out]
        n211 = case shown="False" w340 {
          tunnel: [T20."Enabled" ("Disabled") T20."Disabled and Grayed Out" ("Disabled")] -> w339
          frame False {
          }
          frame True {
          }
        }
        n212 = property on="Single I/Q Capture" class="Bool (strict)"("DisabledEnum"=w339) -> ()  [unwired: 2 in, 2 out]
        n213 = property on="FlexSDR Selection" class="Ring (strict)"("DisabledEnum"=w339) -> ()  [unwired: 2 in, 2 out]
        n214 = property on="Perform CAL" class="Bool (strict)"("DisabledEnum"=w339) -> ()  [unwired: 2 in, 2 out]
      }
      event "Set Default Scale": Value Change {
        n215 = event-data() -> ("NewVal"=w343:bool)  [unwired: 1 in, 5 out]
        n216 = case shown="True" w343 {
          frame False {
          }
          frame True {
            n217 = flat-sequence {
              frame #0 {
                n218 = property on="FFT Mag" class="XYGraph (strict)"("YScale.Maximum"=0.0 ("Y Scale.Range:Maximum"), "YScale.Minimum"=-160.0 ("Y Scale.Range:Minimum"), "XScale.Maximum"=737.28 ("X Scale.Range:Maximum"), "XScale.Minimum"=-737.28 ("X Scale.Range:Minimum")) -> ()  [unwired: 2 in, 2 out]
                n219 = call "Time Delay27"("Delay Time (s)"=0.1) -> ()  [unwired: 10 in, 1 out]
              }
              frame #1 {
                n220 = local write "Set Default Scale"(FALSE ("Set Default Scale")) -> ()
              }
            }
          }
        }
      }
      event "Get Device\nInformation": Value Change {
        n221 = event-data() -> ("NewVal"=w352:bool)  [unwired: 1 in, 5 out]
        n222 = flat-sequence {
          tunnel: w352 -> [w355]
          tunnel: [w355] -> w351
          tunnel: T4 {"reply_information"="", "manufacturer"="", "model"="", "serial_number"=0, "firmware_revision"=""} ("Device\nInformation") -> [w353]
          frame #0 {
            n223 = local write "Device\nInformation"(w353) -> ()
            n224 = local write "Hardware\nBusy"(TRUE ("Hardware\nBusy")) -> ()
          }
        }
        n225 = case shown="True" w351 {
          frame False {
          }
          frame True {
            n226 = local read "FlexSDR Selection"() -> (w367:u16)
            n227 = property on="FlexSDR Selection" class="Ring (strict)"() -> ("Strings []"=w368:string[])  [unwired: 2 in, 2 out]
            n228 = Index Array(array=w368, index=w367) -> (element=w356:string)
            n229 = call "Create Client.vi"("address"=w356) -> ("error out"=w366:errorcluster, "gRPC ID Out"=w365:T45)  [unwired: 9 in]
            n230 = call "RFController GetDeviceInformation.vi"("error in"=w366, "timeout (ms)"=250, "Request Data"=T24 {"device_id"="", "error_queue_populate"=FALSE}, "gRPC ID"=w365) -> ("error out"=w364:errorcluster, "Response Data"=w360:T4, "gRPC ID out"=w363:T45)  [unwired: 5 in]
            n231 = call "Destroy Client.vi"("error in"=w364, "gRPC ID"=w363) -> ("error out"=w359:errorcluster)  [unwired: 9 in]
            n232 = flat-sequence {
              tunnel: w360 -> [w371]
              tunnel: [w371] -> w361
              tunnel: w359 -> [w369]
              tunnel: [w369] -> w358
              tunnel: w361 -> [w374]
              tunnel: w358 -> [w372]
              frame #0 {
                n233 = call "Time Delay3"("Delay Time (s)"=0.25) -> ()  [unwired: 10 in, 1 out]
              }
              frame #1 {
                n234 = local write "Hardware\nBusy"(FALSE ("Hardware\nBusy")) -> ()
                n235 = local write "Get Device\nInformation"(FALSE ("Get Device\nInformation")) -> ()
                n236 = local write "Error Out"(w372) -> ()
                "Device\nInformation" <- w374
              }
            }
          }
        }
      }
      event "Get Center\nFrequency": Value Change {
        n237 = event-data() -> ("NewVal"=w378:bool)  [unwired: 1 in, 5 out]
        n238 = flat-sequence {
          tunnel: w378 -> [w381]
          tunnel: [w381] -> w377
          tunnel: T5 {"center_frequency"=0.0, "error_status"=-1, "error_message"=""} ("Center Frequency Data") -> [w379]
          frame #0 {
            n239 = local write "Center Frequency Data"(w379) -> ()
            n240 = local write "Hardware\nBusy"(TRUE ("Hardware\nBusy")) -> ()
          }
        }
        n241 = case shown="True" w377 {
          frame False {
          }
          frame True {
            (unwired) 250 ("timeout (ms)")
            n242 = local read "FlexSDR Selection"() -> (w394:u16)
            n243 = local read "CF RFDC"() -> (w382:T2)
            n244 = property on="FlexSDR Selection" class="Ring (strict)"() -> ("Strings []"=w395:string[])  [unwired: 2 in, 2 out]
            n245 = Bundle By Name(cluster=T26 {"device_id"="", "rfdc"=enum."TX1", "error_queue_populate"=FALSE} ("Request Data"), "rfdc"=w382) -> (w383:T26)
            n246 = Index Array(array=w395, index=w394) -> (element=w391:string)
            n247 = call "Create Client.vi"("address"=w391) -> ("error out"=w390:errorcluster, "gRPC ID Out"=w389:T45)  [unwired: 9 in]
            n248 = call "RFController GetRFDCCenterFrequency.vi"("error in"=w390, "Request Data"=w383, "gRPC ID"=w389) -> ("error out"=w388:errorcluster, "Response Data"=w386:T5, "gRPC ID out"=w387:T45)  [unwired: 6 in]
            n249 = call "Destroy Client.vi"("error in"=w388, "gRPC ID"=w387) -> ("error out"=w393:errorcluster)  [unwired: 9 in]
            n250 = flat-sequence {
              tunnel: w393 -> [w397]
              tunnel: [w397] -> w392
              tunnel: w386 -> [w396]
              tunnel: [w396] -> w385
              tunnel: w392 -> [w400]
              tunnel: w385 -> [w399]
              frame #0 {
                n251 = call "Time Delay4"("Delay Time (s)"=0.25) -> ()  [unwired: 10 in, 1 out]
              }
              frame #1 {
                n252 = local write "Get Center\nFrequency"(FALSE ("Get Device\nInformation")) -> ()
                n253 = local write "Hardware\nBusy"(FALSE ("Hardware\nBusy")) -> ()
                n254 = local write "Error Out"(w400) -> ()
                "Center Frequency Data" <- w399
              }
            }
          }
        }
      }
      event "Get Gain": Value Change {
        n255 = event-data() -> ("NewVal"=w405:bool)  [unwired: 1 in, 5 out]
        n256 = flat-sequence {
          tunnel: w405 -> [w408]
          tunnel: [w408] -> w404
          tunnel: T6 {"gain"=0.0, "error_status"=-1, "error_message"=""} ("Gain Data") -> [w406]
          frame #0 {
            n257 = local write "Hardware\nBusy"(TRUE ("Hardware\nBusy")) -> ()
            n258 = local write "Gain Data"(w406) -> ()
          }
        }
        n259 = case shown="True" w404 {
          frame False {
          }
          frame True {
            n260 = local read "FlexSDR Selection"() -> (w422:u16)
            n261 = local read "Gain RFDC"() -> (w411:T2)
            n262 = property on="FlexSDR Selection" class="Ring (strict)"() -> ("Strings []"=w423:string[])  [unwired: 2 in, 2 out]
            n263 = Index Array(array=w423, index=w422) -> (element=w419:string)
            n264 = Bundle By Name(cluster=T27 {"device_id"="", "rfdc"=enum."TX1", "error_queue_populate"=FALSE} ("Request Data"), "rfdc"=w411) -> (w412:T27)
            n265 = call "Create Client.vi"("address"=w419) -> ("error out"=w418:errorcluster, "gRPC ID Out"=w417:T45)  [unwired: 9 in]
            n266 = call "RFController GetRFDCGain.vi"("error in"=w418, "timeout (ms)"=250, "Request Data"=w412, "gRPC ID"=w417) -> ("error out"=w416:errorcluster, "Response Data"=w410:T6, "gRPC ID out"=w415:T45)  [unwired: 5 in]
            n267 = call "Destroy Client.vi"("error in"=w416, "gRPC ID"=w415) -> ("error out"=w421:errorcluster)  [unwired: 9 in]
            n268 = flat-sequence {
              tunnel: w421 -> [w425]
              tunnel: [w425] -> w420
              tunnel: w410 -> [w424]
              tunnel: [w424] -> w409
              tunnel: w420 -> [w428]
              tunnel: w409 -> [w427]
              frame #0 {
                n269 = call "Time Delay5"("Delay Time (s)"=0.25) -> ()  [unwired: 10 in, 1 out]
              }
              frame #1 {
                n270 = local write "Hardware\nBusy"(FALSE ("Hardware\nBusy")) -> ()
                n271 = local write "Get Gain"(FALSE ("Get Device\nInformation")) -> ()
                n272 = local write "Error Out"(w428) -> ()
                "Gain Data" <- w427
              }
            }
          }
        }
      }
      event "Get Sample\nRate": Value Change {
        n273 = event-data() -> ("NewVal"=w433:bool)  [unwired: 1 in, 5 out]
        n274 = flat-sequence {
          tunnel: w433 -> [w436]
          tunnel: [w436] -> w432
          tunnel: T8 {"sample_rate"=0.0, "error_status"=-1, "error_message"=""} ("Sample Rate Data") -> [w434]
          frame #0 {
            n275 = local write "Sample Rate Data"(w434) -> ()
            n276 = local write "Hardware\nBusy"(TRUE ("Hardware\nBusy")) -> ()
          }
        }
        n277 = case shown="True" w432 {
          frame False {
          }
          frame True {
            n278 = local read "FlexSDR Selection"() -> (w450:u16)
            n279 = local read "SR RFTile"() -> (w439:T7)
            n280 = property on="FlexSDR Selection" class="Ring (strict)"() -> ("Strings []"=w451:string[])  [unwired: 2 in, 2 out]
            n281 = Index Array(array=w451, index=w450) -> (element=w447:string)
            n282 = Bundle By Name(cluster=T28 {"device_id"="", "rftile"=enum."TXT1", "error_queue_populate"=FALSE} ("Request Data"), "rftile"=w439) -> (w440:T28)
            n283 = call "Create Client.vi"("address"=w447) -> ("error out"=w446:errorcluster, "gRPC ID Out"=w445:T45)  [unwired: 9 in]
            n284 = call "RFController GetRFTileSampleRate.vi"("error in"=w446, "timeout (ms)"=250, "Request Data"=w440, "gRPC ID"=w445) -> ("error out"=w444:errorcluster, "Response Data"=w438:T8, "gRPC ID out"=w443:T45)  [unwired: 5 in]
            n285 = call "Destroy Client.vi"("error in"=w444, "gRPC ID"=w443) -> ("error out"=w449:errorcluster)  [unwired: 9 in]
            n286 = flat-sequence {
              tunnel: w449 -> [w453]
              tunnel: [w453] -> w448
              tunnel: w438 -> [w452]
              tunnel: [w452] -> w437
              tunnel: w448 -> [w456]
              tunnel: w437 -> [w455]
              frame #0 {
                n287 = call "Time Delay6"("Delay Time (s)"=0.25) -> ()  [unwired: 10 in, 1 out]
              }
              frame #1 {
                n288 = local write "Hardware\nBusy"(FALSE ("Hardware\nBusy")) -> ()
                n289 = local write "Get Sample\nRate"(FALSE ("Get Device\nInformation")) -> ()
                n290 = local write "Error Out"(w456) -> ()
                "Sample Rate Data" <- w455
              }
            }
          }
        }
      }
      event "Get Temps": Value Change {
        n291 = event-data() -> ("NewVal"=w461:bool)  [unwired: 1 in, 5 out]
        n292 = flat-sequence {
          tunnel: w461 -> [w464]
          tunnel: [w464] -> w460
          tunnel: T9 {"temp_readings"={"PL_temp"=0.0, "APU_temp"=0.0, "RPU_temp"=0.0}, "error_status"=-1, "error_message"=""} ("Device Temp Data") -> [w462]
          frame #0 {
            n293 = local write "Device Temp Data"(w462) -> ()
            n294 = local write "Hardware\nBusy"(TRUE ("Hardware\nBusy")) -> ()
          }
        }
        n295 = case shown="True" w460 {
          frame False {
          }
          frame True {
            n296 = local read "FlexSDR Selection"() -> (w476:u16)
            n297 = property on="FlexSDR Selection" class="Ring (strict)"() -> ("Strings []"=w477:string[])  [unwired: 2 in, 2 out]
            n298 = Index Array(array=w477, index=w476) -> (element=w473:string)
            n299 = call "Create Client.vi"("address"=w473) -> ("error out"=w472:errorcluster, "gRPC ID Out"=w471:T45)  [unwired: 9 in]
            n300 = call "RFController GetDeviceTemps.vi"("error in"=w472, "timeout (ms)"=5000, "Request Data"=T29 {"device_id"="", "error_queue_populate"=FALSE}, "gRPC ID"=w471) -> ("error out"=w470:errorcluster, "Response Data"=w466:T9, "gRPC ID out"=w469:T45)  [unwired: 5 in]
            n301 = call "Destroy Client.vi"("error in"=w470, "gRPC ID"=w469) -> ("error out"=w475:errorcluster)  [unwired: 9 in]
            n302 = flat-sequence {
              tunnel: w475 -> [w479]
              tunnel: [w479] -> w474
              tunnel: w466 -> [w478]
              tunnel: [w478] -> w465
              tunnel: w474 -> [w482]
              tunnel: w465 -> [w481]
              frame #0 {
                n303 = call "Time Delay18"("Delay Time (s)"=0.25) -> ()  [unwired: 10 in, 1 out]
              }
              frame #1 {
                n304 = local write "Get Temps"(FALSE ("Get Device\nInformation")) -> ()
                n305 = local write "Hardware\nBusy"(FALSE ("Hardware\nBusy")) -> ()
                n306 = local write "Error Out"(w482) -> ()
                "Device Temp Data" <- w481
              }
            }
          }
        }
      }
      event "Set Center\nFrequency": Value Change {
        n307 = event-data() -> ("NewVal"=w487:bool)  [unwired: 1 in, 5 out]
        n308 = flat-sequence {
          tunnel: w487 -> [w490]
          tunnel: [w490] -> w486
          tunnel: T11 {"center_frequency"=0.0, "error_status"=-1, "error_message"=""} ("Response Data") -> [w488]
          frame #0 {
            n309 = local write "SCF Data"(w488) -> ()
            n310 = local write "Hardware\nBusy"(TRUE ("Hardware\nBusy")) -> ()
          }
        }
        n311 = case shown="True" w486 {
          frame False {
          }
          frame True {
            n312 = local read "FlexSDR Selection"() -> (w505:u16)
            n313 = local read "SCF RFDC"() -> (w501:T2)
            n314 = property on="FlexSDR Selection" class="Ring (strict)"() -> ("Strings []"=w506:string[])  [unwired: 2 in, 2 out]
            n315 = Bundle By Name(cluster=T30 {"device_id"="", "rfdc"=enum."TX1", "center_frequency"=0.0, "error_queue_populate"=FALSE} ("Request Data"), "rfdc"=w501, "center_frequency"="Req CF") -> (w491:T30)
            n316 = Index Array(array=w506, index=w505) -> (element=w502:string)
            n317 = call "Create Client.vi"("address"=w502) -> ("error out"=w500:errorcluster, "gRPC ID Out"=w499:T45)  [unwired: 9 in]
            n318 = call "RFController SetRFDCCenterFrequency.vi"("error in"=w500, "timeout (ms)"=5000, "Request Data"=w491, "gRPC ID"=w499) -> ("error out"=w497:errorcluster, "Response Data"=w496:T11, "gRPC ID out"=w498:T45)  [unwired: 5 in]
            n319 = call "Destroy Client.vi"("error in"=w497, "gRPC ID"=w498) -> ("error out"=w504:errorcluster)  [unwired: 9 in]
            n320 = flat-sequence {
              tunnel: w504 -> [w508]
              tunnel: [w508] -> w503
              tunnel: w496 -> [w507]
              tunnel: [w507] -> w495
              tunnel: w503 -> [w511]
              tunnel: w495 -> [w510]
              frame #0 {
                n321 = call "Time Delay7"("Delay Time (s)"=0.25) -> ()  [unwired: 10 in, 1 out]
              }
              frame #1 {
                n322 = local write "Set Center\nFrequency"(FALSE ("Get Device\nInformation")) -> ()
                n323 = local write "Hardware\nBusy"(FALSE ("Hardware\nBusy")) -> ()
                n324 = local write "Error Out"(w511) -> ()
                "SCF Data" <- w510
              }
            }
          }
        }
      }
      event "Set Gain": Value Change {
        n325 = event-data() -> ("NewVal"=w516:bool)  [unwired: 1 in, 5 out]
        n326 = flat-sequence {
          tunnel: w516 -> [w519]
          tunnel: [w519] -> w515
          tunnel: T12 {"gain"=0.0, "error_status"=-1, "error_message"=""} ("SG Data") -> [w517]
          frame #0 {
            n327 = local write "SG Data"(w517) -> ()
            n328 = local write "Hardware\nBusy"(TRUE ("Hardware\nBusy")) -> ()
          }
        }
        n329 = case shown="True" w515 {
          frame False {
          }
          frame True {
            n330 = local read "FlexSDR Selection"() -> (w534:u16)
            n331 = local read "SG RFDC"() -> (w530:T2)
            n332 = property on="FlexSDR Selection" class="Ring (strict)"() -> ("Strings []"=w535:string[])  [unwired: 2 in, 2 out]
            n333 = Index Array(array=w535, index=w534) -> (element=w531:string)
            n334 = Bundle By Name(cluster=T31 {"device_id"="", "rfdc"=enum."TX1", "gain"=0.0, "error_queue_populate"=FALSE} ("Request Data"), "rfdc"=w530, "gain"="Req Gain") -> (w520:T31)
            n335 = call "Create Client.vi"("address"=w531) -> ("error out"=w529:errorcluster, "gRPC ID Out"=w528:T45)  [unwired: 9 in]
            n336 = call "RFController SetRFDCGain.vi"("error in"=w529, "timeout (ms)"=5000, "Request Data"=w520, "gRPC ID"=w528) -> ("error out"=w527:errorcluster, "Response Data"=w525:T12, "gRPC ID out"=w526:T45)  [unwired: 5 in]
            n337 = call "Destroy Client.vi"("error in"=w527, "gRPC ID"=w526) -> ("error out"=w533:errorcluster)  [unwired: 9 in]
            n338 = flat-sequence {
              tunnel: w533 -> [w537]
              tunnel: [w537] -> w532
              tunnel: w525 -> [w536]
              tunnel: [w536] -> w524
              tunnel: w532 -> [w540]
              tunnel: w524 -> [w539]
              frame #0 {
                n339 = call "Time Delay8"("Delay Time (s)"=0.25) -> ()  [unwired: 10 in, 1 out]
              }
              frame #1 {
                n340 = local write "Hardware\nBusy"(FALSE ("Hardware\nBusy")) -> ()
                n341 = local write "Error Out"(w540) -> ()
                n342 = local write "Set Gain"(FALSE ("Get Device\nInformation")) -> ()
                "SG Data" <- w539
              }
            }
          }
        }
      }
      event "Set Sample\nRate": Value Change {
        n343 = event-data() -> ("NewVal"=w545:bool)  [unwired: 1 in, 5 out]
        n344 = flat-sequence {
          tunnel: w545 -> [w548]
          tunnel: [w548] -> w544
          tunnel: T13 {"sample_rate"=0.0, "error_status"=-1, "error_message"=""} ("SSR Data") -> [w546]
          frame #0 {
            n345 = local write "SSR Data"(w546) -> ()
            n346 = local write "Hardware\nBusy"(TRUE ("Hardware\nBusy")) -> ()
          }
        }
        n347 = case shown="True" w544 {
          frame False {
          }
          frame True {
            n348 = local read "FlexSDR Selection"() -> (w563:u16)
            n349 = local read "SSR RFTile"() -> (w559:T7)
            n350 = property on="FlexSDR Selection" class="Ring (strict)"() -> ("Strings []"=w564:string[])  [unwired: 2 in, 2 out]
            n351 = Bundle By Name(cluster=T32 {"device_id"="", "rftile"=enum."TXT1", "sample_rate"=0.0, "error_queue_populate"=FALSE} ("Request Data"), "rftile"=w559, "sample_rate"="Req SR") -> (w551:T32)
            n352 = Index Array(array=w564, index=w563) -> (element=w560:string)
            n353 = call "Create Client.vi"("address"=w560) -> ("error out"=w558:errorcluster, "gRPC ID Out"=w556:T45)  [unwired: 9 in]
            n354 = call "RFController SetRFTileSampleRate.vi"("error in"=w558, "timeout (ms)"=5000, "Request Data"=w551, "gRPC ID"=w556) -> ("error out"=w557:errorcluster, "Response Data"=w550:T13, "gRPC ID out"=w555:T45)  [unwired: 5 in]
            n355 = call "Destroy Client.vi"("error in"=w557, "gRPC ID"=w555) -> ("error out"=w562:errorcluster)  [unwired: 9 in]
            n356 = flat-sequence {
              tunnel: w562 -> [w566]
              tunnel: [w566] -> w561
              tunnel: w550 -> [w565]
              tunnel: [w565] -> w549
              tunnel: w561 -> [w569]
              tunnel: w549 -> [w568]
              frame #0 {
                n357 = call "Time Delay9"("Delay Time (s)"=0.25) -> ()  [unwired: 10 in, 1 out]
              }
              frame #1 {
                n358 = local write "Hardware\nBusy"(FALSE ("Hardware\nBusy")) -> ()
                n359 = local write "Error Out"(w569) -> ()
                n360 = local write "Set Sample\nRate"(FALSE ("Get Device\nInformation")) -> ()
                "SSR Data" <- w568
              }
            }
          }
        }
      }
      event "Perform CAL": Value Change {
        n361 = event-data() -> ("NewVal"=w573:bool)  [unwired: 1 in, 5 out]
        n362 = flat-sequence {
          tunnel: w573 -> [w581]
          tunnel: [w581] -> w572
          frame #0 {
            w574 = FALSE ("Grabbing\n100 MHz")
            w576 = 0.0 ("Full BW EVM")
            w575 = FALSE ("Analyzing\nFull BW")
            n363 = call "Build XY Graph6"("Reset"=TRUE) -> ("XY Graph"=w579:cluster{"X":dbl[], "Y":dbl[]}[])  [unwired: 9 in, 1 out]
            n364 = local write "Grabbing\nFull BW"(TRUE ("Grabbing\nFull BW")) -> ()
            n365 = local write "Analyzing\nFull BW"(w575) -> ()
            n366 = local write "Writing \nCal Coeffs"(w575) -> ()
            n367 = local write "Grabbing\n1200 MHz"(w575) -> ()
            n368 = local write "Analyzing\n1200 MHz"(w575) -> ()
            n369 = local write "Grabbing\n400 MHz"(w575) -> ()
            n370 = local write "Analyzing\n400 MHz"(w575) -> ()
            n371 = local write "Hardware\nBusy"(TRUE ("Hardware\nBusy")) -> ()
            n372 = local write "Cal FFT Mag"(w579) -> ()
            n373 = local write "Grabbing\n100 MHz"(w574) -> ()
            n374 = local write "Analyzing\n100 MHz"(w574) -> ()
            n375 = local write "Complete"(w574) -> ()
            n376 = local write "Full BW EVM"(w576) -> ()
            n377 = local write "1200 EVM"(w576) -> ()
            n378 = local write "400 EVM"(w576) -> ()
            n379 = local write "100 EVM"(w576) -> ()
          }
        }
        n380 = case shown="True" w572 {
          frame False {
          }
          frame True {
            w630 = "calibration_1200_full" ("waveform_type")
            w617 = 61440 ("num_of_samples")
            w625 = 10000 ("timeout (ms)")
            n381 = local read "FlexSDR Selection"() -> (w649:u16)
            n382 = property on="FlexSDR Selection" class="Ring (strict)"() -> ("Strings []"=w650:string[])  [unwired: 2 in, 2 out]
            n383 = Index Array(array=w650, index=w649) -> (element=w648:string)
            n384 = call "Create Client.vi"("address"=w648) -> ("error out"=w646:errorcluster, "gRPC ID Out"=w645:T45)  [unwired: 9 in]
            n385 = call "RFController GetRFDCBackgroundCalibrationState.vi"("error in"=w646, "timeout (ms)"=w625, "Request Data"=T35 {"device_id"="", "rfdc"=enum."WRX1", "error_queue_populate"=FALSE}, "gRPC ID"=w645) -> ("error out"=w629:errorcluster, "Response Data"=w643:T14, "gRPC ID out"=w628:T45)  [unwired: 5 in]
            n386 = call "RFController SetRFDCCalibrationBypass.vi"("error in"=w629, "timeout (ms)"=w625, "Request Data"=T33 {"device_id"="", "rfdc"=enum."WRX1", "bypass_cal"=TRUE, "error_queue_populate"=FALSE}, "gRPC ID"=w628) -> ("error out"=w627:errorcluster, "Response Data"=w623:T17, "gRPC ID out"=w626:T45)  [unwired: 5 in]
            n387 = flat-sequence {
              tunnel: w623 -> [_]
              frame #0 {
              }
            }
            n388 = call "Calibraiton_Procedure.vi"("timeout (ms)"=w625, "error in"=w627, "num_of_samples"=w617, "waveform_type"=w630, "gRPC ID in"=w626) -> ("error out"=w638:errorcluster, "Response Data"=w637:T46, "gRPC ID out"=w634:T45)
            n389 = call "IQ_Data_Processing.vi"("file name"="Full_BW_Pre_Cal.csv", "WFM Capture Response"=w637, "error in"=w638) -> ("FFT Mag XY"=w635:cluster{"X":dbl[], "Y":dbl[]}[], "error out"=w631:errorcluster)  [unwired: 3 out]
            n390 = local read "Show Matlab"() -> (w612:bool)
            n391 = local write "Cal FFT Mag"(w635) -> ()
            n392 = local read "Cal Level"() -> (w620:dbl)
            n393 = flat-sequence {
              tunnel: w634 -> [w661]
              tunnel: w631 -> [w660]
              tunnel: w630 -> [w659]
              tunnel: [w661] -> w622
              tunnel: [w660] -> w621
              tunnel: w620 -> [w655]
              tunnel: w617 -> [w656]
              tunnel: [w656] -> w616
              tunnel: w612 -> [w654]
              tunnel: [w655] -> w611
              tunnel: [w654] -> w609
              tunnel: w622 -> [w669]
              tunnel: w621 -> [w668]
              tunnel: [w666] -> w619
              tunnel: [w667] -> w618
              tunnel: w616 -> [w664]
              tunnel: [w664] -> w615
              tunnel: w611 -> [w663]
              tunnel: [w663] -> w610
              tunnel: w609 -> [w662]
              tunnel: [w662] -> w608
              tunnel: w619 -> [w681]
              tunnel: w618 -> [w682]
              tunnel: w615 -> [w671]
              tunnel: [w680] -> w614
              tunnel: [w678] -> w613
              tunnel: w610 -> [w672]
              tunnel: w608 -> [w673]
              tunnel: [w673] -> w607
              tunnel: [w672] -> w606
              tunnel: [w671] -> w605
              tunnel: [w670] -> w604
              tunnel: w614 -> [w693]
              tunnel: w613 -> [w692]
              tunnel: w607 -> [w688]
              tunnel: w606 -> [w689]
              tunnel: w605 -> [w691]
              tunnel: w604 -> [w690]
              tunnel: [w693] -> w603
              tunnel: [w692] -> w602
              tunnel: [w688] -> w601
              tunnel: [w689] -> w600
              tunnel: [w691] -> w599
              tunnel: w603 -> [w700]
              tunnel: w602 -> [w701]
              tunnel: w601 -> [w706]
              tunnel: w600 -> [w705]
              tunnel: w599 -> [w699]
              tunnel: [w697] -> w598
              tunnel: [w698] -> w597
              tunnel: [w706] -> w596
              tunnel: [w705] -> w595
              tunnel: [w699] -> w594
              tunnel: [w694] -> w593
              tunnel: w598 -> [w717]
              tunnel: w597 -> [w716]
              tunnel: w596 -> [w712]
              tunnel: w595 -> [w713]
              tunnel: w594 -> [w715]
              tunnel: w593 -> [w714]
              tunnel: [w717] -> w592
              tunnel: [w716] -> w591
              tunnel: [w712] -> w590
              tunnel: [w713] -> w589
              tunnel: [w715] -> w588
              tunnel: w592 -> [w725]
              tunnel: w591 -> [w724]
              tunnel: w590 -> [w730]
              tunnel: w589 -> [w729]
              tunnel: w588 -> [w718]
              tunnel: [w723] -> w587
              tunnel: [w722] -> w586
              tunnel: [w730] -> w585
              tunnel: [w729] -> w584
              tunnel: [w718] -> w583
              tunnel: [w719] -> w582
              tunnel: [w739] -> _
              tunnel: [w737] -> _
              tunnel: [w736] -> _
              tunnel: [w740] -> w632
              tunnel: [w741] -> w633
              tunnel: w587 -> [w741]
              tunnel: w586 -> [w740]
              tunnel: w585 -> [w736]
              tunnel: w584 -> [w737]
              tunnel: w583 -> [w739]
              tunnel: w582 -> [w738]
              frame #0 {
                w651 = 800.0 ("X Scale.Range:Maximum")
                n394 = call "Run_Calibration_Matlab.vi"("Show Matlab"=w654, "Cal Level"=w655, "Selection String"=w659) -> ("EVM Post-Cal"=w657:dbl)  [unwired: 1 in, 1 out]
                n395 = Negate(x=w651) -> (-x=w653:dbl)
                n396 = local write "Analyzing\nFull BW"(TRUE ("Analyzing\nFull BW")) -> ()
                n397 = local write "Full BW EVM"(w657) -> ()
                n398 = property on="Cal FFT Mag" class="XYGraph (strict)"("XScale.Maximum"=w651, "XScale.Minimum"=w653, "YScale.Minimum"=-70.0 ("Y Scale.Range:Minimum")) -> ()  [unwired: 2 in, 2 out]
              }
              frame #1 {
                n399 = local write "Writing \nCal Coeffs"(TRUE ("Writing \nCal Coeffs")) -> ()
                n400 = call "Write_EQ_and_Enable.vi"("error in"=w668, "gRPC ID in"=w669) -> ("error out"=w667:errorcluster, "gRPC ID out"=w666:T45)  [unwired: 2 in, 2 out]
              }
              frame #2 {
                w670 = "calibration_1200" ("waveform_type")
                n401 = local write "Grabbing\n1200 MHz"(TRUE ("Grabbing\n1200 MHz")) -> ()
                n402 = call "Calibraiton_Procedure.vi"("error in"=w682, "num_of_samples"=w671, "waveform_type"=w670, "gRPC ID in"=w681) -> ("error out"=w679:errorcluster, "Response Data"=w677:T46, "gRPC ID out"=w680:T45)  [unwired: 1 in]
                n403 = call "IQ_Data_Processing.vi"("file name"="1200_MHz_Post_Cal.csv", "WFM Capture Response"=w677, "error in"=w679) -> ("FFT Mag XY"=w675:cluster{"X":dbl[], "Y":dbl[]}[], "error out"=w678:errorcluster)  [unwired: 3 out]
                n404 = local write "Cal FFT Mag"(w675) -> ()
              }
              frame #3 {
                w684 = 650.0 ("X Scale.Range:Maximum")
                n405 = local write "Analyzing\n1200 MHz"(TRUE ("Analyzing\n1200 MHz")) -> ()
                n406 = call "Run_Calibration_Matlab.vi"("Show Matlab"=w688, "Cal Level"=w689, "Selection String"=w690) -> ("EVM Pre-Cal"=w687:dbl)  [unwired: 1 in, 1 out]
                n407 = Negate(x=w684) -> (-x=w685:dbl)
                n408 = property on="Cal FFT Mag" class="XYGraph (strict)"("XScale.Maximum"=w684, "XScale.Minimum"=w685, "YScale.Minimum"=-130.0 ("Y Scale.Range:Minimum")) -> ()  [unwired: 2 in, 2 out]
                n409 = local write "1200 EVM"(w687) -> ()
              }
              frame #4 {
                w694 = "calibration_400" ("waveform_type")
                n410 = local write "Grabbing\n400 MHz"(TRUE ("Grabbing\n400 MHz")) -> ()
                n411 = call "Calibraiton_Procedure.vi"("error in"=w701, "num_of_samples"=w699, "waveform_type"=w694, "gRPC ID in"=w700) -> ("error out"=w704:errorcluster, "Response Data"=w703:T46, "gRPC ID out"=w697:T45)  [unwired: 1 in]
                n412 = call "IQ_Data_Processing.vi"("file name"="400_MHz_Post_Cal.csv", "WFM Capture Response"=w703, "error in"=w704) -> ("FFT Mag XY"=w695:cluster{"X":dbl[], "Y":dbl[]}[], "error out"=w698:errorcluster)  [unwired: 3 out]
                n413 = local write "Cal FFT Mag"(w695) -> ()
              }
              frame #5 {
                w708 = 220.0 ("X Scale.Range:Maximum")
                n414 = call "Run_Calibration_Matlab.vi"("Show Matlab"=w712, "Cal Level"=w713, "Selection String"=w714) -> ("EVM Pre-Cal"=w711:dbl)  [unwired: 1 in, 1 out]
                n415 = Negate(x=w708) -> (-x=w709:dbl)
                n416 = local write "Analyzing\n400 MHz"(TRUE ("Analyzing\n400 MHz")) -> ()
                n417 = property on="Cal FFT Mag" class="XYGraph (strict)"("XScale.Maximum"=w708, "XScale.Minimum"=w709, "YScale.Minimum"=-130.0 ("Y Scale.Range:Minimum")) -> ()  [unwired: 2 in, 2 out]
                n418 = local write "400 EVM"(w711) -> ()
              }
              frame #6 {
                w719 = "calibration_100" ("waveform_type")
                n419 = local write "Grabbing\n100 MHz"(TRUE ("Grabbing\n100 MHz")) -> ()
                n420 = call "Calibraiton_Procedure.vi"("error in"=w724, "num_of_samples"=w718, "waveform_type"=w719, "gRPC ID in"=w725) -> ("error out"=w728:errorcluster, "Response Data"=w727:T46, "gRPC ID out"=w723:T45)  [unwired: 1 in]
                n421 = call "IQ_Data_Processing.vi"("file name"="100_MHz_Post_Cal.csv", "WFM Capture Response"=w727, "error in"=w728) -> ("FFT Mag XY"=w720:cluster{"X":dbl[], "Y":dbl[]}[], "error out"=w722:errorcluster)  [unwired: 3 out]
                n422 = local write "Cal FFT Mag"(w720) -> ()
              }
              frame #7 {
                w732 = 55.0 ("X Scale.Range:Maximum")
                n423 = call "Run_Calibration_Matlab.vi"("Show Matlab"=w736, "Cal Level"=w737, "Selection String"=w738) -> ("EVM Pre-Cal"=w735:dbl)  [unwired: 1 in, 1 out]
                n424 = local write "Analyzing\n100 MHz"(TRUE ("Analyzing\n100 MHz")) -> ()
                n425 = Negate(x=w732) -> (-x=w733:dbl)
                n426 = local write "100 EVM"(w735) -> ()
                n427 = property on="Cal FFT Mag" class="XYGraph (strict)"("XScale.Maximum"=w732, "XScale.Minimum"=w733, "YScale.Minimum"=-130.0 ("Y Scale.Range:Minimum")) -> ()  [unwired: 2 in, 2 out]
              }
            }
            n428 = Unbundle By Name(w643) -> ("is_frozen"=w642:bool)
            n429 = case shown="False" w642 {
              tunnel: w632 -> [w746 w747]
              tunnel: w633 -> [w745 w748]
              tunnel: [w743 w748] -> w641
              tunnel: [w744 w747] -> w640
              tunnel: T34 {"device_id"="", "rfdc"=enum."WRX1", "is_frozen"=FALSE, "error_queue_populate"=FALSE} ("Request Data") -> [w742 _]
              frame False {
                n430 = call "RFController SetRFDCBackgroundCalibrationState.vi"("error in"=w746, "Request Data"=w742, "gRPC ID"=w745) -> ("error out"=w744:errorcluster, "gRPC ID out"=w743:T45)  [unwired: 6 in, 1 out]
              }
              frame True {
              }
            }
            n431 = call "Destroy Client.vi"("error in"=w640, "gRPC ID"=w641) -> ("error out"=w647:errorcluster)  [unwired: 9 in]
            n432 = flat-sequence {
              tunnel: w647 -> [w750]
              frame #0 {
                n433 = local write "Hardware\nBusy"(FALSE ("Hardware\nBusy")) -> ()
                n434 = local write "Perform CAL"(FALSE ("Get Device\nInformation")) -> ()
                n435 = local write "Complete"(TRUE ("Complete")) -> ()
                n436 = local write "Error Out"(w750) -> ()
              }
            }
          }
        }
      }
      event "Get BGCal\nStatus": Value Change {
        n437 = event-data() -> ("NewVal"=w755:bool)  [unwired: 1 in, 5 out]
        n438 = flat-sequence {
          tunnel: w755 -> [w758]
          tunnel: [w758] -> w754
          tunnel: T14 {"is_frozen"=FALSE, "error_status"=-1, "error_message"=""} ("BGCal Data") -> [w756]
          frame #0 {
            n439 = local write "BGCal Data"(w756) -> ()
            n440 = local write "Hardware\nBusy"(TRUE ("Hardware\nBusy")) -> ()
          }
        }
        n441 = case shown="True" w754 {
          frame False {
          }
          frame True {
            n442 = local read "FlexSDR Selection"() -> (w772:u16)
            n443 = local read "BGCal RFDC"() -> (w768:T2)
            n444 = property on="FlexSDR Selection" class="Ring (strict)"() -> ("Strings []"=w773:string[])  [unwired: 2 in, 2 out]
            n445 = Index Array(array=w773, index=w772) -> (element=w769:string)
            n446 = Bundle By Name(cluster=T35 {"device_id"="", "rfdc"=enum."TX1", "error_queue_populate"=FALSE} ("Request Data"), "rfdc"=w768) -> (w761:T35)
            n447 = call "Create Client.vi"("address"=w769) -> ("error out"=w767:errorcluster, "gRPC ID Out"=w766:T45)  [unwired: 9 in]
            n448 = call "RFController GetRFDCBackgroundCalibrationState.vi"("error in"=w767, "timeout (ms)"=250, "Request Data"=w761, "gRPC ID"=w766) -> ("error out"=w765:errorcluster, "Response Data"=w760:T14, "gRPC ID out"=w764:T45)  [unwired: 5 in]
            n449 = call "Destroy Client.vi"("error in"=w765, "gRPC ID"=w764) -> ("error out"=w771:errorcluster)  [unwired: 9 in]
            n450 = flat-sequence {
              tunnel: w771 -> [w775]
              tunnel: [w775] -> w770
              tunnel: w760 -> [w774]
              tunnel: [w774] -> w759
              tunnel: w770 -> [w778]
              tunnel: w759 -> [w777]
              frame #0 {
                n451 = call "Time Delay10"("Delay Time (s)"=0.25) -> ()  [unwired: 10 in, 1 out]
              }
              frame #1 {
                n452 = local write "Get BGCal\nStatus"(FALSE ("Get Device\nInformation")) -> ()
                n453 = local write "Hardware\nBusy"(FALSE ("Hardware\nBusy")) -> ()
                n454 = local write "Error Out"(w778) -> ()
                "BGCal Data" <- w777
              }
            }
          }
        }
      }
      event "Set BGCal\nStatus": Value Change {
        n455 = event-data() -> ("NewVal"=w783:bool)  [unwired: 1 in, 5 out]
        n456 = flat-sequence {
          tunnel: w783 -> [w786]
          tunnel: [w786] -> w782
          tunnel: T15 {"is_frozen"=FALSE, "error_status"=-1, "error_message"=""} ("SBGCal Data") -> [w784]
          frame #0 {
            n457 = local write "SBGCal Data"(w784) -> ()
            n458 = local write "Hardware\nBusy"(TRUE ("Hardware\nBusy")) -> ()
          }
        }
        n459 = case shown="True" w782 {
          frame False {
          }
          frame True {
            n460 = local read "New Frozen\nStatus"() -> (w790:bool)
            n461 = local read "FlexSDR Selection"() -> (w801:u16)
            n462 = local read "SBGCal RFDC"() -> (w797:T2)
            n463 = property on="FlexSDR Selection" class="Ring (strict)"() -> ("Strings []"=w802:string[])  [unwired: 2 in, 2 out]
            n464 = Index Array(array=w802, index=w801) -> (element=w798:string)
            n465 = Bundle By Name(cluster=T34 {"device_id"="", "rfdc"=enum."TX1", "is_frozen"=FALSE, "error_queue_populate"=FALSE} ("Request Data"), "rfdc"=w797, "is_frozen"=w790) -> (w789:T34)
            n466 = call "Create Client.vi"("address"=w798) -> ("error out"=w796:errorcluster, "gRPC ID Out"=w795:T45)  [unwired: 9 in]
            n467 = call "RFController SetRFDCBackgroundCalibrationState.vi"("error in"=w796, "timeout (ms)"=5000, "Request Data"=w789, "gRPC ID"=w795) -> ("error out"=w794:errorcluster, "Response Data"=w788:T15, "gRPC ID out"=w793:T45)  [unwired: 5 in]
            n468 = call "Destroy Client.vi"("error in"=w794, "gRPC ID"=w793) -> ("error out"=w800:errorcluster)  [unwired: 9 in]
            n469 = flat-sequence {
              tunnel: w800 -> [w804]
              tunnel: [w804] -> w799
              tunnel: w788 -> [w803]
              tunnel: [w803] -> w787
              tunnel: w799 -> [w807]
              tunnel: w787 -> [w806]
              frame #0 {
                n470 = call "Time Delay11"("Delay Time (s)"=0.25) -> ()  [unwired: 10 in, 1 out]
              }
              frame #1 {
                n471 = local write "Hardware\nBusy"(FALSE ("Hardware\nBusy")) -> ()
                n472 = local write "Error Out"(w807) -> ()
                n473 = local write "Set BGCal\nStatus"(FALSE ("Get Device\nInformation")) -> ()
                "SBGCal Data" <- w806
              }
            }
          }
        }
      }
      event "Get Cal\nStatus": Value Change {
        n474 = event-data() -> ("NewVal"=w812:bool)  [unwired: 1 in, 5 out]
        n475 = flat-sequence {
          tunnel: w812 -> [w815]
          tunnel: [w815] -> w811
          tunnel: T16 {"bypass_cal"=FALSE, "error_status"=-1, "error_message"=""} ("Cal Status Data") -> [w813]
          frame #0 {
            n476 = local write "Cal Status Data"(w813) -> ()
            n477 = local write "Hardware\nBusy"(TRUE ("Hardware\nBusy")) -> ()
          }
        }
        n478 = case shown="True" w811 {
          frame False {
          }
          frame True {
            n479 = local read "FlexSDR Selection"() -> (w829:u16)
            n480 = local read "Cal RFDC"() -> (w825:T2)
            n481 = property on="FlexSDR Selection" class="Ring (strict)"() -> ("Strings []"=w830:string[])  [unwired: 2 in, 2 out]
            n482 = Index Array(array=w830, index=w829) -> (element=w826:string)
            n483 = Bundle By Name(cluster=T36 {"device_id"="", "rfdc"=enum."TX1", "error_queue_populate"=FALSE} ("Request Data"), "rfdc"=w825) -> (w818:T36)
            n484 = call "Create Client.vi"("address"=w826) -> ("error out"=w824:errorcluster, "gRPC ID Out"=w821:T45)  [unwired: 9 in]
            n485 = call "RFController GetRFDCCalibrationBypass.vi"("error in"=w824, "timeout (ms)"=250, "Request Data"=w818, "gRPC ID"=w821) -> ("error out"=w823:errorcluster, "Response Data"=w817:T16, "gRPC ID out"=w822:T45)  [unwired: 5 in]
            n486 = call "Destroy Client.vi"("error in"=w823, "gRPC ID"=w822) -> ("error out"=w828:errorcluster)  [unwired: 9 in]
            n487 = flat-sequence {
              tunnel: w828 -> [w832]
              tunnel: [w832] -> w827
              tunnel: w817 -> [w831]
              tunnel: [w831] -> w816
              tunnel: w827 -> [w835]
              tunnel: w816 -> [w834]
              frame #0 {
                n488 = call "Time Delay12"("Delay Time (s)"=0.25) -> ()  [unwired: 10 in, 1 out]
              }
              frame #1 {
                n489 = local write "Hardware\nBusy"(FALSE ("Hardware\nBusy")) -> ()
                n490 = local write "Get Cal\nStatus"(FALSE ("Get Device\nInformation")) -> ()
                n491 = local write "Error Out"(w835) -> ()
                "Cal Status Data" <- w834
              }
            }
          }
        }
      }
      event "Set Cal\nStatus": Value Change {
        n492 = event-data() -> ("NewVal"=w840:bool)  [unwired: 1 in, 5 out]
        n493 = flat-sequence {
          tunnel: w840 -> [w843]
          tunnel: [w843] -> w839
          tunnel: T17 {"bypass_cal"=FALSE, "error_status"=-1, "error_message"=""} ("SCal Status Data") -> [w841]
          frame #0 {
            n494 = local write "SCal Status Data"(w841) -> ()
            n495 = local write "Hardware\nBusy"(TRUE ("Hardware\nBusy")) -> ()
          }
        }
        n496 = case shown="True" w839 {
          frame False {
          }
          frame True {
            n497 = local read "FlexSDR Selection"() -> (w858:u16)
            n498 = local read "New Cal Status"() -> (w847:bool)
            n499 = local read "SBCal RFDC"() -> (w854:T2)
            n500 = property on="FlexSDR Selection" class="Ring (strict)"() -> ("Strings []"=w859:string[])  [unwired: 2 in, 2 out]
            n501 = Bundle By Name(cluster=T33 {"device_id"="", "rfdc"=enum."TX1", "bypass_cal"=FALSE, "error_queue_populate"=FALSE} ("Request Data"), "rfdc"=w854, "bypass_cal"=w847) -> (w846:T33)
            n502 = Index Array(array=w859, index=w858) -> (element=w855:string)
            n503 = call "Create Client.vi"("address"=w855) -> ("error out"=w853:errorcluster, "gRPC ID Out"=w852:T45)  [unwired: 9 in]
            n504 = call "RFController SetRFDCCalibrationBypass.vi"("error in"=w853, "timeout (ms)"=5000, "Request Data"=w846, "gRPC ID"=w852) -> ("error out"=w850:errorcluster, "Response Data"=w845:T17, "gRPC ID out"=w851:T45)  [unwired: 5 in]
            n505 = call "Destroy Client.vi"("error in"=w850, "gRPC ID"=w851) -> ("error out"=w857:errorcluster)  [unwired: 9 in]
            n506 = flat-sequence {
              tunnel: w857 -> [w861]
              tunnel: [w861] -> w856
              tunnel: w845 -> [w860]
              tunnel: [w860] -> w844
              tunnel: w856 -> [w864]
              tunnel: w844 -> [w863]
              frame #0 {
                n507 = call "Time Delay13"("Delay Time (s)"=0.25) -> ()  [unwired: 10 in, 1 out]
              }
              frame #1 {
                n508 = local write "Hardware\nBusy"(FALSE ("Hardware\nBusy")) -> ()
                n509 = local write "Error Out"(w864) -> ()
                n510 = local write "Set Cal\nStatus"(FALSE ("Get Device\nInformation")) -> ()
                "SCal Status Data" <- w863
              }
            }
          }
        }
      }
      event "Get Trig\nStatus": Value Change {
        n511 = event-data() -> ("NewVal"=w868:bool)  [unwired: 1 in, 5 out]
        n512 = flat-sequence {
          tunnel: w868 -> [w874]
          tunnel: [w874] -> w867
          frame #0 {
            w871 = 0 ("Trig Delay")
            w872 = FALSE ("Triggered?")
            n513 = local write "Get Trig Status Error Message"("" ("Get Trig Status Error Message")) -> ()
            n514 = local write "Hardware\nBusy"(TRUE ("Hardware\nBusy")) -> ()
            n515 = local write "Trig Max Length"(w871) -> ()
            n516 = local write "Get Trig Status Error Status"(-1 ("Get Trig Status Error Status")) -> ()
            n517 = local write "Triggered?"(w872) -> ()
            n518 = local write "Wait For Trig?"(w872) -> ()
            n519 = local write "Hardware Trig?"(w872) -> ()
            n520 = local write "Trig Delay"(w871) -> ()
          }
        }
        n521 = case shown="True" w867 {
          frame False {
          }
          frame True {
            n522 = local read "FlexSDR Selection"() -> (w889:u16)
            n523 = local read "Channel #"() -> (w880:i32)
            n524 = local read "Quad #"() -> (w879:i32)
            n525 = property on="FlexSDR Selection" class="Ring (strict)"() -> ("Strings []"=w890:string[])  [unwired: 2 in, 2 out]
            n526 = Bundle By Name(cluster=T37 {"device_id"="", "quad_num"=0, "channel_num"=0, "error_queue_populate"=FALSE} ("Request Data"), "quad_num"=w879, "channel_num"=w880) -> (w878:T37)
            n527 = Index Array(array=w890, index=w889) -> (element=w886:string)
            n528 = call "Create Client.vi"("address"=w886) -> ("error out"=w885:errorcluster, "gRPC ID Out"=w884:T45)  [unwired: 9 in]
            n529 = call "RFController GetTriggerStatus.vi"("error in"=w885, "timeout (ms)"=5000, "Request Data"=w878, "gRPC ID"=w884) -> ("error out"=w883:errorcluster, "Response Data"=w876:T47, "gRPC ID out"=w882:T45)  [unwired: 5 in]
            n530 = call "Destroy Client.vi"("error in"=w883, "gRPC ID"=w882) -> ("error out"=w888:errorcluster)  [unwired: 9 in]
            n531 = flat-sequence {
              tunnel: w888 -> [w892]
              tunnel: [w892] -> w887
              tunnel: w876 -> [w891]
              tunnel: [w891] -> w875
              tunnel: w887 -> [w902]
              tunnel: w875 -> [w901]
              frame #0 {
                n532 = call "Time Delay14"("Delay Time (s)"=0.25) -> ()  [unwired: 10 in, 1 out]
              }
              frame #1 {
                n533 = local write "Hardware\nBusy"(FALSE ("Hardware\nBusy")) -> ()
                n534 = local write "Get Trig\nStatus"(FALSE ("Get Device\nInformation")) -> ()
                n535 = local write "Error Out"(w902) -> ()
                n536 = Unbundle By Name(w901) -> ("triggered"=w900:bool, "wait_for_trig"=w899:bool, "trig_sample_delay"=w898:i32, "is_hardware_trig"=w897:bool, "max_trig_length"=w896:i32, "error_status"=w895:i32, "error_message"=w894:string)  [unwired: 2 out]
                n537 = local write "Triggered?"(w900) -> ()
                n538 = local write "Wait For Trig?"(w899) -> ()
                n539 = local write "Trig Delay"(w898) -> ()
                n540 = local write "Hardware Trig?"(w897) -> ()
                n541 = local write "Trig Max Length"(w896) -> ()
                n542 = local write "Get Trig Status Error Status"(w895) -> ()
                n543 = local write "Get Trig Status Error Message"(w894) -> ()
              }
            }
          }
        }
      }
      event "Set Trig Wait": Value Change {
        n544 = event-data() -> ("NewVal"=w906:bool)  [unwired: 1 in, 5 out]
        n545 = flat-sequence {
          tunnel: w906 -> [w910]
          tunnel: [w910] -> w905
          frame #0 {
            n546 = local write "Set Trig Wait Error Message"("" ("Set Trig Wait Error Message")) -> ()
            n547 = local write "Set Trig Wait Error Status"(-1 ("Set Trig Wait Error Status")) -> ()
            n548 = local write "Hardware\nBusy"(TRUE ("Hardware\nBusy")) -> ()
          }
        }
        n549 = case shown="True" w905 {
          frame False {
          }
          frame True {
            n550 = local read "Set Hardware Trig"() -> (w911:bool)
            n551 = local read "FlexSDR Selection"() -> (w927:u16)
            n552 = local read "Set Trig Delay"() -> (w912:i32)
            n553 = local read "Channel #"() -> (w915:i32)
            n554 = local read "Quad #"() -> (w916:i32)
            n555 = property on="FlexSDR Selection" class="Ring (strict)"() -> ("Strings []"=w928:string[])  [unwired: 2 in, 2 out]
            n556 = Bundle By Name(cluster=T38 {"device_id"="", "quad_num"=0, "channel_num"=0, "trig_sample_delay"=0, "is_hardware_trig"=FALSE, "error_queue_populate"=FALSE} ("Request Data"), "quad_num"=w916, "channel_num"=w915, "trig_sample_delay"=w912, "is_hardware_trig"=w911) -> (w917:T38)
            n557 = Index Array(array=w928, index=w927) -> (element=w924:string)
            n558 = call "Create Client.vi"("address"=w924) -> ("error out"=w923:errorcluster, "gRPC ID Out"=w922:T45)  [unwired: 9 in]
            n559 = call "RFController SetTriggerWait.vi"("error in"=w923, "timeout (ms)"=5000, "Request Data"=w917, "gRPC ID"=w922) -> ("error out"=w921:errorcluster, "Response Data"=w914:T48, "gRPC ID out"=w920:T45)  [unwired: 5 in]
            n560 = call "Destroy Client.vi"("error in"=w921, "gRPC ID"=w920) -> ("error out"=w926:errorcluster)  [unwired: 9 in]
            n561 = flat-sequence {
              tunnel: w926 -> [w930]
              tunnel: [w930] -> w925
              tunnel: w914 -> [w929]
              tunnel: [w929] -> w913
              tunnel: w925 -> [w935]
              tunnel: w913 -> [w934]
              frame #0 {
                n562 = call "Time Delay15"("Delay Time (s)"=0.25) -> ()  [unwired: 10 in, 1 out]
              }
              frame #1 {
                n563 = local write "Hardware\nBusy"(FALSE ("Hardware\nBusy")) -> ()
                n564 = local write "Error Out"(w935) -> ()
                n565 = local write "Set Trig Wait"(FALSE ("Get Device\nInformation")) -> ()
                n566 = Unbundle By Name(w934) -> ("error_status"=w933:i32, "error_message"=w932:string)
                n567 = local write "Set Trig Wait Error Message"(w932) -> ()
                n568 = local write "Set Trig Wait Error Status"(w933) -> ()
              }
            }
          }
        }
      }
      event "Set Trig Max Length": Value Change {
        n569 = event-data() -> ("NewVal"=w939:bool)  [unwired: 1 in, 5 out]
        n570 = flat-sequence {
          tunnel: w939 -> [w943]
          tunnel: [w943] -> w938
          frame #0 {
            n571 = local write "Set Trig Max Length Error Status"(-1 ("Set Trig Wait Error Status")) -> ()
            n572 = local write "Set Trig Max Length Error Message"("" ("Set Trig Wait Error Message")) -> ()
            n573 = local write "Hardware\nBusy"(TRUE ("Hardware\nBusy")) -> ()
          }
        }
        n574 = case shown="True" w938 {
          frame False {
          }
          frame True {
            n575 = local read "Set Trig Max Length Value"() -> (w945:i32)
            n576 = local read "FlexSDR Selection"() -> (w959:u16)
            n577 = property on="FlexSDR Selection" class="Ring (strict)"() -> ("Strings []"=w960:string[])  [unwired: 2 in, 2 out]
            n578 = local read "Channel #"() -> (w954:i32)
            n579 = local read "Quad #"() -> (w955:i32)
            n580 = Index Array(array=w960, index=w959) -> (element=w956:string)
            n581 = Bundle By Name(cluster=T39 {"device_id"="", "quad_num"=0, "channel_num"=0, "max_trig_length"=0, "error_queue_populate"=FALSE} ("Request Data"), "quad_num"=w955, "channel_num"=w954, "max_trig_length"=w945) -> (w944:T39)
            n582 = call "Create Client.vi"("address"=w956) -> ("error out"=w953:errorcluster, "gRPC ID Out"=w951:T45)  [unwired: 9 in]
            n583 = call "RFController SetMaxTriggerLength.vi"("error in"=w953, "timeout (ms)"=5000, "Request Data"=w944, "gRPC ID"=w951) -> ("error out"=w952:errorcluster, "Response Data"=w949:T49, "gRPC ID out"=w950:T45)  [unwired: 5 in]
            n584 = call "Destroy Client.vi"("error in"=w952, "gRPC ID"=w950) -> ("error out"=w958:errorcluster)  [unwired: 9 in]
            n585 = flat-sequence {
              tunnel: w958 -> [w962]
              tunnel: [w962] -> w957
              tunnel: w949 -> [w961]
              tunnel: [w961] -> w948
              tunnel: w957 -> [w967]
              tunnel: w948 -> [w964]
              frame #0 {
                n586 = call "Time Delay17"("Delay Time (s)"=0.25) -> ()  [unwired: 10 in, 1 out]
              }
              frame #1 {
                n587 = local write "Hardware\nBusy"(FALSE ("Hardware\nBusy")) -> ()
                n588 = local write "Set Trig Max Length"(FALSE ("Get Device\nInformation")) -> ()
                n589 = local write "Error Out"(w967) -> ()
                n590 = Unbundle By Name(w964) -> ("error_status"=w966:i32, "error_message"=w965:string)
                n591 = local write "Set Trig Wait Error Message"(w965) -> ()
                n592 = local write "Set Trig Wait Error Status"(w966) -> ()
              }
            }
          }
        }
      }
      event "Reset Trig": Value Change {
        n593 = event-data() -> ("NewVal"=w971:bool)  [unwired: 1 in, 5 out]
        n594 = flat-sequence {
          tunnel: w971 -> [w975]
          tunnel: [w975] -> w970
          frame #0 {
            n595 = local write "Reset Trig Error Message"("" ("Set Trig Wait Error Message")) -> ()
            n596 = local write "Reset Trig Error Status"(-1 ("Set Trig Wait Error Status")) -> ()
            n597 = local write "Hardware\nBusy"(TRUE ("Hardware\nBusy")) -> ()
          }
        }
        n598 = case shown="True" w970 {
          frame False {
          }
          frame True {
            n599 = local read "FlexSDR Selection"() -> (w990:u16)
            n600 = local read "Channel #"() -> (w979:i32)
            n601 = local read "Quad #"() -> (w980:i32)
            n602 = property on="FlexSDR Selection" class="Ring (strict)"() -> ("Strings []"=w991:string[])  [unwired: 2 in, 2 out]
            n603 = Bundle By Name(cluster=T40 {"device_id"="", "quad_num"=0, "channel_num"=0, "error_queue_populate"=FALSE} ("Request Data"), "quad_num"=w980, "channel_num"=w979) -> (w978:T40)
            n604 = Index Array(array=w991, index=w990) -> (element=w987:string)
            n605 = call "Create Client.vi"("address"=w987) -> ("error out"=w986:errorcluster, "gRPC ID Out"=w983:T45)  [unwired: 9 in]
            n606 = call "RFController ResetTrigger.vi"("error in"=w986, "timeout (ms)"=5000, "Request Data"=w978, "gRPC ID"=w983) -> ("error out"=w985:errorcluster, "Response Data"=w977:T50, "gRPC ID out"=w984:T45)  [unwired: 5 in]
            n607 = call "Destroy Client.vi"("error in"=w985, "gRPC ID"=w984) -> ("error out"=w989:errorcluster)  [unwired: 9 in]
            n608 = flat-sequence {
              tunnel: w989 -> [w993]
              tunnel: [w993] -> w988
              tunnel: w977 -> [w992]
              tunnel: [w992] -> w976
              tunnel: w988 -> [w998]
              tunnel: w976 -> [w995]
              frame #0 {
                n609 = call "Time Delay16"("Delay Time (s)"=0.25) -> ()  [unwired: 10 in, 1 out]
              }
              frame #1 {
                n610 = local write "Hardware\nBusy"(FALSE ("Hardware\nBusy")) -> ()
                n611 = local write "Reset Trig"(FALSE ("Get Device\nInformation")) -> ()
                n612 = local write "Error Out"(w998) -> ()
                n613 = Unbundle By Name(w995) -> ("error_status"=w997:i32, "error_message"=w996:string)
                n614 = local write "Reset Trig Error Status"(w997) -> ()
                n615 = local write "Reset Trig Error Message"(w996) -> ()
              }
            }
          }
        }
      }
      event "Start GPS \nPoll": Value Change {
        n616 = event-data() -> ("NewVal"=w1002:bool)  [unwired: 1 in, 5 out]
        n617 = flat-sequence {
          tunnel: w1002 -> [w1006]
          tunnel: [w1003] -> w1001
          frame #0 {
            n618 = local read "GPS Poll Active"() -> (w1005:bool)
            n619 = local write "Hardware\nBusy"(TRUE ("Hardware\nBusy")) -> ()
            n620 = Not(x=w1005) -> (.not. x?=w1004:bool)
            n621 = And(x=w1006, y=w1004) -> (x .and. y?=w1003:bool)
          }
        }
        n622 = case shown="True" w1001 {
          frame False {
          }
          frame True {
            n623 = local read "FlexSDR Selection"() -> (w1019:u16)
            n624 = property on="FlexSDR Selection" class="Ring (strict)"() -> ("Strings []"=w1020:string[])  [unwired: 2 in, 2 out]
            n625 = Index Array(array=w1020, index=w1019) -> (element=w1016:string)
            n626 = call "Create Client.vi"("address"=w1016) -> ("error out"=w1015:errorcluster, "gRPC ID Out"=w1014:T45)  [unwired: 9 in]
            n627 = call "RFController StartGPSPoll.vi"("error in"=w1015, "Request Data"=T41 {"device_id"="", "error_queue_populate"=FALSE}, "gRPC ID"=w1014) -> ("error out"=w1013:errorcluster, "Response Data"=w1008:T51, "gRPC ID out"=w1012:T45)  [unwired: 6 in]
            n628 = property on="Stop Program" class="Bool (strict)"("DisabledEnum"=T20."Disabled and Grayed Out" ("Disabled")) -> ()  [unwired: 2 in, 2 out]
            n629 = call "Destroy Client.vi"("error in"=w1013, "gRPC ID"=w1012) -> ("error out"=w1018:errorcluster)  [unwired: 9 in]
            n630 = flat-sequence {
              tunnel: w1018 -> [w1027]
              tunnel: [w1027] -> w1017
              tunnel: w1008 -> [w1026]
              tunnel: [w1025] -> w1010
              tunnel: w1017 -> [w1031]
              tunnel: w1010 -> [w1029]
              frame #0 {
                n631 = Unbundle By Name(w1026) -> ("gps_poll_status"=w1024:bool, "error_status"=w1023:i32)
                n632 = call "Time Delay19"("Delay Time (s)"=0.25) -> ()  [unwired: 10 in, 1 out]
                n633 = Equal?(x=w1023, y=0) -> (x = y?=w1021:bool)
                n634 = And(x=w1024, y=w1021) -> (x .and. y?=w1025:bool)
              }
              frame #1 {
                n635 = case shown="True" w1029 {
                  frame False {
                  }
                  frame True {
                    n636 = local write "GPS Poll Active"(TRUE ("GPS Poll Active")) -> ()
                  }
                }
                n637 = local write "Hardware\nBusy"(FALSE ("Hardware\nBusy")) -> ()
                n638 = local write "Start GPS \nPoll"(FALSE ("Get Device\nInformation")) -> ()
                n639 = local write "Error Out"(w1031) -> ()
              }
            }
          }
        }
      }
      event "Stop GPS\nPoll": Value Change {
        n640 = event-data() -> ("NewVal"=w1035:bool)  [unwired: 1 in, 5 out]
        n641 = flat-sequence {
          tunnel: w1035 -> [w1038]
          tunnel: [w1037] -> w1034
          frame #0 {
            n642 = local read "GPS Poll Active"() -> (w1036:bool)
            n643 = local write "Hardware\nBusy"(TRUE ("Hardware\nBusy")) -> ()
            n644 = And(x=w1038, y=w1036) -> (x .and. y?=w1037:bool)
          }
        }
        n645 = case shown="True" w1034 {
          frame False {
          }
          frame True {
            n646 = local read "FlexSDR Selection"() -> (w1051:u16)
            n647 = property on="FlexSDR Selection" class="Ring (strict)"() -> ("Strings []"=w1052:string[])  [unwired: 2 in, 2 out]
            n648 = Index Array(array=w1052, index=w1051) -> (element=w1048:string)
            n649 = call "Create Client.vi"("address"=w1048) -> ("error out"=w1045:errorcluster, "gRPC ID Out"=w1041:T45)  [unwired: 9 in]
            n650 = call "RFController StopGPSPoll.vi"("error in"=w1045, "Request Data"=T42 {"device_id"="", "error_queue_populate"=FALSE}, "gRPC ID"=w1041) -> ("error out"=w1044:errorcluster, "Response Data"=w1042:T52, "gRPC ID out"=w1043:T45)  [unwired: 6 in]
            n651 = property on="Stop Program" class="Bool (strict)"("DisabledEnum"=T20."Enabled" ("Disabled")) -> ()  [unwired: 2 in, 2 out]
            n652 = call "Destroy Client.vi"("error in"=w1044, "gRPC ID"=w1043) -> ("error out"=w1050:errorcluster)  [unwired: 9 in]
            n653 = flat-sequence {
              tunnel: w1050 -> [w1060]
              tunnel: [w1060] -> w1049
              tunnel: w1042 -> [w1059]
              tunnel: [w1058] -> w1047
              tunnel: w1049 -> [w1064]
              tunnel: w1047 -> [w1062]
              frame #0 {
                n654 = Unbundle By Name(w1059) -> ("gps_poll_status"=w1053:bool, "error_status"=w1057:i32)
                n655 = call "Time Delay21"("Delay Time (s)"=0.25) -> ()  [unwired: 10 in, 1 out]
                n656 = Equal?(x=w1057, y=0) -> (x = y?=w1055:bool)
                n657 = Not(x=w1053) -> (.not. x?=w1054:bool)
                n658 = And(x=w1054, y=w1055) -> (x .and. y?=w1058:bool)
              }
              frame #1 {
                n659 = case shown="False" w1062 {
                  frame False {
                  }
                  frame True {
                    n660 = local write "GPS Poll Active"(FALSE ("GPS Poll Active")) -> ()
                  }
                }
                n661 = local write "Hardware\nBusy"(FALSE ("Hardware\nBusy")) -> ()
                n662 = local write "Stop GPS\nPoll"(FALSE ("Get Device\nInformation")) -> ()
                n663 = local write "Error Out"(w1064) -> ()
              }
            }
          }
        }
      }
      event "Set UTC\nStart Time": Value Change {
        n664 = event-data() -> ("NewVal"=w1068:bool)  [unwired: 1 in, 5 out]
        n665 = flat-sequence {
          tunnel: w1068 -> [w1069]
          tunnel: [w1069] -> w1067
          frame #0 {
            n666 = local write "Hardware\nBusy"(TRUE ("Hardware\nBusy")) -> ()
          }
        }
        n667 = case shown="True" w1067 {
          frame False {
          }
          frame True {
            n668 = local read "FlexSDR Selection"() -> (w1083:u16)
            n669 = local read "UTC Start Time"() -> (w1071:dbl)
            n670 = property on="FlexSDR Selection" class="Ring (strict)"() -> ("Strings []"=w1084:string[])  [unwired: 2 in, 2 out]
            n671 = Bundle By Name(cluster=T43 {"device_id"="", "utc_start_time"=0.0, "error_queue_populate"=FALSE} ("Request Data"), "utc_start_time"=w1071) -> (w1074:T43)
            n672 = Index Array(array=w1084, index=w1083) -> (element=w1080:string)
            n673 = call "Create Client.vi"("address"=w1080) -> ("error out"=w1079:errorcluster, "gRPC ID Out"=w1078:T45)  [unwired: 9 in]
            n674 = call "RFController SetGPSUTCStartTime.vi"("error in"=w1079, "Request Data"=w1074, "gRPC ID"=w1078) -> ("error out"=w1077:errorcluster, "Response Data"=w1073:T18, "gRPC ID out"=w1076:T45)  [unwired: 6 in]
            n675 = call "Destroy Client.vi"("error in"=w1077, "gRPC ID"=w1076) -> ("error out"=w1082:errorcluster)  [unwired: 9 in]
            n676 = flat-sequence {
              tunnel: w1082 -> [w1086]
              tunnel: [w1086] -> w1081
              tunnel: w1073 -> [w1085]
              tunnel: [w1085] -> w1072
              tunnel: w1081 -> [w1090]
              tunnel: w1072 -> [w1088]
              frame #0 {
                n677 = call "Time Delay23"("Delay Time (s)"=0.25) -> ()  [unwired: 10 in, 1 out]
              }
              frame #1 {
                n678 = local write "Hardware\nBusy"(FALSE ("Hardware\nBusy")) -> ()
                n679 = local write "Set UTC\nStart Time"(FALSE ("Get Device\nInformation")) -> ()
                n680 = local write "Error Out"(w1090) -> ()
                "UTS Start Time Response" <- w1088
              }
            }
          }
        }
      }
      event "Main Container": Value Change {
        n681 = event-data() -> ("OldVal"=w1095:T1)  [unwired: 1 in, 5 out]
        n682 = local read "GPS Poll Active"() -> (w1093:bool)
        n683 = local read "KPI Poll"() -> (w1094:bool)
        n684 = Or(x=w1094, y=w1093) -> (x .or. y?=w1092:bool)
        n685 = case shown="True" w1092 {
          tunnel: w1095 -> [_ w1096]
          frame False {
          }
          frame True {
            n686 = property on="Main Container" class="TabCtl (strict)"("Value"=w1096) -> ()  [unwired: 2 in, 2 out]
          }
        }
      }
      event "Update Server\nControls": Value Change {
        n687 = event-data() -> ("NewVal"=w1099:bool)  [unwired: 1 in, 5 out]
        n688 = flat-sequence {
          tunnel: w1099 -> [w1101]
          tunnel: [w1101] -> w1098
          tunnel: T19 {"message"=""} ("Update Server Controls Response") -> [w1100]
          frame #0 {
            n689 = local write "Update Server Controls Response"(w1100) -> ()
            n690 = local write "Hardware\nBusy"(TRUE ("Hardware\nBusy")) -> ()
          }
        }
        n691 = case shown="True" w1098 {
          frame False {
          }
          frame True {
            n692 = local read "Set Time Between Peaks"() -> (w1107:dbl)
            n693 = local read "Set Server Sample Rate"() -> (w1110:dbl)
            n694 = local read "Set Carrier Frequency"() -> (w1109:dbl)
            n695 = local read "Set Peak Threshold"() -> (w1111:dbl)
            n696 = local read "Set Sync Length"() -> (w1108:i32)
            n697 = Multiply(x=w1107, y=122.88) -> (x*y=w1105:dbl)
            n698 = local read "FlexCompute Selection"() -> (w1121:u16)
            n699 = Bundle By Name(cluster=T44 {"peak_threshold"=0.0, "sampling_rate_hz"=0.0, "carrier_frequency_hz"=0.0, "sync_length_samples"=0, "time_between_peaks_s"=0.0} ("Request Data"), "peak_threshold"=w1111, "sampling_rate_hz"=w1110, "carrier_frequency_hz"=w1109, "sync_length_samples"=w1108, "time_between_peaks_s"=w1105) -> (w1112:T44)
            n700 = property on="FlexCompute Selection" class="Ring (strict)"() -> ("Strings []"=w1122:string[])  [unwired: 2 in, 2 out]
            n701 = Index Array(array=w1122, index=w1121) -> (element=w1120:string)
            n702 = call "Create Client.vi"("address"=w1120) -> ("error out"=w1119:errorcluster, "gRPC ID Out"=w1118:T45)  [unwired: 9 in]
            n703 = call "RFController setDPDKKPIControlParams.vi"("error in"=w1119, "Request Data"=w1112, "gRPC ID"=w1118) -> ("error out"=w1117:errorcluster, "Response Data"=w1104:T19, "gRPC ID out"=w1116:T45)  [unwired: 6 in]
            n704 = call "Destroy Client.vi"("error in"=w1117, "gRPC ID"=w1116) -> ("error out"=w1114:errorcluster)  [unwired: 9 in]
            n705 = flat-sequence {
              tunnel: w1114 -> [w1124]
              tunnel: [w1124] -> w1113
              tunnel: w1104 -> [w1123]
              tunnel: [w1123] -> w1103
              tunnel: w1113 -> [w1127]
              tunnel: w1103 -> [w1126]
              frame #0 {
                n706 = call "Time Delay20"("Delay Time (s)"=0.25) -> ()  [unwired: 10 in, 1 out]
              }
              frame #1 {
                n707 = local write "Hardware\nBusy"(FALSE ("Hardware\nBusy")) -> ()
                n708 = local write "Update Server\nControls"(FALSE ("Get Device\nInformation")) -> ()
                n709 = local write "Error Out"(w1127) -> ()
                "Update Server Controls Response" <- w1126
              }
            }
          }
        }
      }
    }
    n710 = Subtract(x=w99, y=w93) -> (x-y=w92:u32)
    n711 = local read "KPI Poll"() -> (w96:bool)
    n712 = Subtract(x=w99, y=w101) -> (x-y=w102:u32)
    n713 = Greater?(x=w92, y=w98) -> (0:w97:bool)
    n714 = Greater?(x=w102, y=w105) -> (0:w104:bool)
    n715 = And(x=w96, y=w97) -> (x .and. y?=w95:bool)
    n716 = And(x=w106, y=w104) -> (x .and. y?=w103:bool)
    n717 = case shown="True" w103 {
      tunnel: [w175 w183] -> w107
      tunnel: w102 -> [_ w176]
      tunnel: w101 -> [w175 _]
      frame False {
      }
      frame True {
        n718 = local write "GPS Actual Poll Time"(w176) -> ()
        n719 = flat-sequence {
          tunnel: [w189] -> w182
          tunnel: [w188] -> w181
          tunnel: [w187] -> w180
          tunnel: [w186] -> w179
          tunnel: [w185] -> w178
          tunnel: [w184] -> w177
          tunnel: [w208] -> w183
          tunnel: w182 -> [w207]
          tunnel: w181 -> [w205]
          tunnel: w180 -> [w204]
          tunnel: w179 -> [w203]
          tunnel: w178 -> [w202]
          tunnel: w177 -> [w201]
          frame #0 {
            n720 = local read "GPS Num of Samples"() -> (w193:i32)
            n721 = local read "FlexSDR Selection"() -> (w199:u16)
            n722 = property on="FlexSDR Selection" class="Ring (strict)"() -> ("Strings []"=w200:string[])  [unwired: 2 in, 2 out]
            n723 = Bundle By Name(cluster=T23 {"device_id"="", "num_of_samples"=0, "error_queue_populate"=FALSE} ("Request Data"), "num_of_samples"=w193) -> (w194:T23)
            n724 = Index Array(array=w200, index=w199) -> (element=w198:string)
            n725 = call "Create Client.vi"("address"=w198) -> ("error out"=w197:errorcluster, "gRPC ID Out"=w196:T45)  [unwired: 9 in]
            n726 = call "RFController GetGPSLastLocInfo.vi"("error in"=w197, "Request Data"=w194, "gRPC ID"=w196) -> ("error out"=w192:errorcluster, "Response Data"=w190:T53, "gRPC ID out"=w191:T45)  [unwired: 6 in]
            n727 = call "Destroy Client.vi"("error in"=w192, "gRPC ID"=w191) -> ()  [unwired: 9 in, 1 out]
            n728 = Unbundle By Name(w190) -> ("time"=w189:dbl[], "ecef_x"=w188:dbl[], "ecef_y"=w187:dbl[], "ecef_z"=w186:dbl[], "error_status"=w184:i32, "error_message"=w185:string)
          }
          frame #1 {
            n729 = local write "GPS ECEF Y"(w204) -> ()
            n730 = local write "GPS ECEF Z"(w203) -> ()
            n731 = local write "GPS ECEF X"(w205) -> ()
            n732 = local write "GPS error_status"(w201) -> ()
            n733 = local write "GPS error_message"(w202) -> ()
            n734 = for {
              tunnel: w207 -> [w211] mode=indexing
              tunnel: [w210] -> w206 mode=indexing
              n735 = local read "Display \nTimestamp?"() -> (w209:bool)
              n736 = case shown="False" w209 {
                tunnel: w211 -> [w214 w220]
                tunnel: [w212 w215] -> w210
                frame False {
                  n737 = Number To Fractional String(number=w214, precision (6)=i16 1) -> (F-format string=w212:string)  [unwired: 2 in]
                }
                frame True {
                  n738 = Add(x=w220, y=2082844800.0) -> (x+y=w219:dbl)
                  n739 = To Time Stamp(1:w219) -> (0:w217:timestamp)
                  n740 = Format Date/Time String(time format string (%c)="%Y/%m/%d %H:%M:%S%1u %Z", seconds (now)=w217, UTC format=TRUE) -> (date/time string=w215:string)
                }
              }
            }
            n741 = local write "GPS Time"(w206) -> ()
            n742 = Tick Count (ms)() -> (millisecond timer value=w208:u32)
          }
        }
      }
    }
    n743 = case shown="False" w95 {
      tunnel: [w110 w123] -> w94
      tunnel: w93 -> [w110 _]
      tunnel: w92 -> [_ w122]
      frame False {
      }
      frame True {
        n744 = local write "Actual KPI Poll Time"(w122) -> ()
        n745 = flat-sequence {
          tunnel: [w134] -> w121
          tunnel: [w133] -> w120
          tunnel: [w132] -> w119
          tunnel: [w131] -> w118
          tunnel: [w130] -> w117
          tunnel: [w129] -> w116
          tunnel: [w128] -> w115
          tunnel: [w127] -> w114
          tunnel: [w126] -> w113
          tunnel: [w125] -> w112
          tunnel: [w124] -> w111
          tunnel: [w154] -> w123
          tunnel: w121 -> [w153]
          tunnel: w120 -> [w152]
          tunnel: w119 -> [w151]
          tunnel: w118 -> [_]
          tunnel: w117 -> [w150]
          tunnel: w116 -> [w147]
          tunnel: w115 -> [w146]
          tunnel: w114 -> [w145]
          tunnel: w113 -> [w144]
          tunnel: w112 -> [w149]
          tunnel: w111 -> [w148]
          frame #0 {
            n746 = local read "FlexCompute Selection"() -> (w142:u16)
            n747 = property on="FlexCompute Selection" class="Ring (strict)"() -> ("Strings []"=w143:string[])  [unwired: 2 in, 2 out]
            n748 = Index Array(array=w143, index=w142) -> (element=w141:string)
            n749 = call "Create Client.vi"("address"=w141) -> ("error out"=w140:errorcluster, "gRPC ID Out"=w139:T45)  [unwired: 9 in]
            n750 = call "RFController getDPDKKPI.vi"("error in"=w140, "Request Data"=T21 {"void"=""}, "gRPC ID"=w139) -> ("error out"=w137:errorcluster, "Response Data"=w135:T54, "gRPC ID out"=w136:T45)  [unwired: 6 in]
            n751 = call "Destroy Client.vi"("error in"=w137, "gRPC ID"=w136) -> ()  [unwired: 9 in, 1 out]
            n752 = Unbundle By Name(w135) -> ("peak_threshold"=w134:dbl, "rssi_db"=w133:dbl, "timing_offset_s"=w132:dbl, "peak_index_samples"=w131:i32, "peak_time_s"=w130:dbl, "is_anomaly"=w129:bool, "mem_address"=w128:string, "status"=w127:T55, "error_message"=w126:string, "phase_rotation_from_peak_I"=w125:sgl, "phase_rotation_from_peak_Q"=w124:sgl)
          }
          frame #1 {
            n753 = Tick Count (ms)() -> (millisecond timer value=w154:u32)
            "RSSI" <- w152
            "Peak Time Offset" <- w151
            "Peak Time" <- w150
            "I Phase Rotation From Peak" <- w149
            "Q Phase Rotation From Peak" <- w148
            "Peak Threshold" <- w153
            "Anomaly \nDetected" <- w147
            "Mem Address" <- w146
            "KPI Status" <- w145
            "KPI Error Message" <- w144
          }
        }
      }
    }
    n754 = local read "Continuous I/Q Capture"() -> (w100:bool)
    n755 = case shown="True" w100 {
      frame False {
      }
      frame True {
        n756 = local read "Capture Length"() -> (w164:i32)
        n757 = local read "FlexSDR Selection"() -> (w165:u16)
        n758 = local read "Capture RFDC"() -> (w163:T2)
        n759 = property on="FlexSDR Selection" class="Ring (strict)"() -> ("Strings []"=w166:string[])  [unwired: 2 in, 2 out]
        n760 = Bundle By Name(cluster=T22 {"device_id"="", "rfdc"=enum."TX1", "num_of_samples"=0, "error_queue_populate"=FALSE} ("Request Data"), "rfdc"=w163, "num_of_samples"=w164) -> (w167:T22)
        n761 = Index Array(array=w166, index=w165) -> (element=w174:string)
        n762 = call "Create Client.vi"("address"=w174) -> ("error out"=w173:errorcluster, "gRPC ID Out"=w172:T45)  [unwired: 9 in]
        n763 = call "RFController RFDCCaptureWaveform.vi"("error in"=w173, "timeout (ms)"=10000, "Request Data"=w167, "gRPC ID"=w172) -> ("error out"=w171:errorcluster, "Response Data"=w161:T46, "gRPC ID out"=w170:T45)  [unwired: 5 in]
        n764 = call "Destroy Client.vi"("error in"=w171, "gRPC ID"=w170) -> ("error out"=w162:errorcluster)  [unwired: 9 in]
        n765 = call "IQ_Data_Processing.vi"("file name"="capture.csv", "WFM Capture Response"=w161, "error in"=w162) -> ("gRPC error_status"=w158:i32, "gRPC error_message"=w157:string, "FFT Mag XY"=w156:cluster{"X":dbl[], "Y":dbl[]}[], "IQ XY"=w155:cluster{"X":dbl[], "Y":dbl[]}[], "error out"=w159:errorcluster)
        n766 = local write "Capture Error Status"(w158) -> ()
        n767 = local write "FFT Mag"(w156) -> ()
        n768 = local write "IQ Graph"(w155) -> ()
        n769 = local write "Capture Error Message"(w157) -> ()
        n770 = local write "Error Out"(w159) -> ()
      }
    }
    n771 = local read "Stop Program"() -> (w109:bool)
  }
  n772 = flat-sequence {
    tunnel: w2 -> [w1131]
    tunnel: [w1131] -> w1
    tunnel: w1 -> [w1133]
    frame #0 {
      n773 = call "Time Delay"("Delay Time (s)"=0.25) -> ()  [unwired: 10 in, 1 out]
    }
    frame #1 {
      n774 = Not(x=w1133) -> (.not. x?=w1132:bool)
      n775 = local write "Stop Program"(w1132) -> ()
    }
  }
